vi "PROGRAM v0.96.vi"() -> ()   [LabVIEW 2015]
uses:
  <vilib>/Analysis/Matrix/Datatypes/RealMatrix.ctl
  <vilib>/DAQmx/write.llb/DAQmx Write (Digital 1D Bool 1Chan 1Samp).vi
  <vilib>/DAQmx/write.llb/DAQmx Write (Digital 1D Bool NChan 1Samp 1Line).vi
  <vilib>/DAQmx/read.llb/DAQmx Read (Analog Wfm 1Chan NSamp).vi
  <vilib>/DAQmx/write.llb/DAQmx Write (Analog 1D DBL NChan 1Samp).vi
  <vilib>/DAQmx/miscellaneous.llb/DAQmx Fill In Error Info.vi
  <vilib>/express/express analysis/Spectral/Block/exnSpectralBlock spectral measurements peak poly.vi
  <vilib>/express/express analysis/Spectral/Block/exnSpectralBlock spectral measurements peak WFM.vi
  <vilib>/express/express analysis/Spectral/XNode/ExpressSpectralMeasurementsBlockNode.xnode
  <vilib>/Analysis/Matrix/NI_Matrix.lvlib
panel:
  in  "Boolean":bool
  out "Kortslutningsström":dbl
  out "EQEvarv 2":i32
  in  "matrix":T1
  in  "Area":dbl caption="Frequency"
  out "Kortslutningsström frekvens":dbl
  in  "EQE-graf":enum32{"Sekvens-graf", "Frekvens-graf"}(tab)
  out "EQE sekvens graf":cluster{dbl[], ext[unit][]}(graph)
  out "EQE frekvens graf":cluster{dbl[], ext[unit][]}(graph)
  in  "stop":bool=TRUE
  in  "Ström från EQE-mätning":dbl[](array[numeric])
  in  "Reglage 720 nm":dbl(slide)=95.45983019683155 scale=0.0..100.0
  in  "Reglage 980 nm":dbl(slide)=100.00009164020905 scale=0.0..100.0
  in  "Reglage 830 nm":dbl(slide)=55.95186186163266 scale=0.0..100.0
  in  "Reglage 590 nm":dbl(slide)=99.99995581432673 scale=0.0..100.0
  in  "Reglage 515 nm":dbl(slide)=34.61040031085785 scale=0.0..100.0
  in  "Reglage 490 nm":dbl(slide)=100.00002446609867 scale=0.0..100.0
  in  "Reglage 750 nm":dbl(slide)=43.28879590477169 scale=0.0..100.0
  in  "Reglage 660 nm":dbl(slide)=45.024171978950314 scale=0.0..100.0
  in  "Reglage 630 nm":dbl(slide)=63.99528760647585 scale=0.0..100.0
  in  "Reglage 780 nm":dbl(slide)=34.69416555258395 scale=0.0..100.0
  in  "Reglage 450 nm":dbl(slide)=50.23408880646861 scale=0.0..100.0
  in  "Reglage 420 nm":dbl(slide)=37.90622795810308 caption="420 nm" scale=0.0..100.0 scale format="%3.0f"
  in  "Reglage 880 nm":dbl(slide)=65.6949904347887 scale=0.0..100.0
  in  "Reglage 945 nm":dbl(slide)=23.435133120769358 scale=0.0..100.0
  in  "Reglage 680 nm":dbl(slide)=85.53036777533312 scale=0.0..100.0
  in  "Reglage 520 nm":dbl(slide)=95.60915775479367 scale=0.0..100.0
  out "Kortslutnings-\nström":dbl
  out "Öppen krets-\nspänning":dbl
  out "PCE":dbl
  out "Fill factor":dbl format="%_6g"
  in  "Avsluta programmet":bool
  in  "Tänd/släck solen":bool
  out "EQEvarv":i32
  in  "Textfil":path
  in  "Val av EQE-mätning":enum32{"Sekvens", "Frekvens"}(radio)
  in  "Fördröjning/punkt (s)":dbl
  in  "Maximal ström":dbl=0.1
  in  "Frekvens (520 nm)":dbl caption="Frequency"
  out "IV-graf":cluster{"Voltage":sgl[], "Current":sgl[]}(graph)
  in  "Area":dbl caption="Frequency"
  in  "EQE-mätning":bool
  in  "IV-mätning":bool
  in  "Steglängd":dbl caption="Frequency"
  in  "Minspänning":dbl caption="Frequency"
  in  "Maxspänning":dbl caption="Frequency"
  in  "Alternativ":u16(ring)=2 items=["Ställ in värden manuellt", "Ställ in värden med reglage", "Standardspektrum AM1.5", "Nollställ alla intensiteter", "Maxa alla intensiteter", "Läs in spektrum från textfil"]
  in  "Intensitet (720)":dbl=40.363
  in  "Intensitet (980)":dbl=88.8364
  in  "Frekvens (720 nm)":dbl caption="Frequency"
  in  "Frekvens (980 nm)":dbl caption="Frequency"
  in  "Intensitet (830)":dbl=46.9522
  in  "Intensitet (590)":dbl=80.0856
  in  "Intensitet (515)":dbl=21.5524
  in  "Frekvens (830 nm)":dbl caption="Frequency"
  in  "Frekvens (590 nm)":dbl caption="Frequency"
  in  "Frekvens (515 nm)":dbl caption="Frequency"
  in  "Intensitet (490)":dbl=48.2735
  in  "Intensitet (750)":dbl=31.2257
  in  "Intensitet (660)":dbl=33.2227
  in  "Frekvens (490 nm)":dbl caption="Frequency"
  in  "Frekvens (750 nm)":dbl caption="Frequency"
  in  "Frekvens (660 nm)":dbl caption="Frequency"
  in  "Intensitet (630)":dbl=48.8157
  in  "Intensitet (780)":dbl=43.738
  in  "Frekvens (630 nm)":dbl caption="Frequency"
  in  "Frekvens (780 nm)":dbl caption="Frequency"
  in  "Intensitet (450)":dbl=50.5233
  in  "Intensitet (420)":dbl=40.9749
  in  "Intensitet (880)":dbl=49.2385
  in  "Frekvens (450 nm)":dbl caption="Frequency"
  in  "Frekvens (420 nm)":dbl caption="Frequency"
  in  "Frekvens (880 nm)":dbl caption="Frequency"
  in  "Intensitet (945)":dbl=21.9074
  in  "Intensitet (680)":dbl=38.1331
  in  "Intensitet (520)":dbl=56.6743
  in  "Andel intensitet för\nangivet spektrum":dbl(slide)=1.0 scale=0.0001..1.0
  in  "Frekvens (945 nm)":dbl caption="Frequency"
  in  "Frekvens (680 nm)":dbl caption="Frequency"
  # "Intensitet"
  # "420 nm"
  # "450 nm"
  # "490 nm"
  # "515 nm"
  # "520 nm"
  # "590 nm"
  # "630 nm"
  # "660 nm"
  # "Intensitet (W/m²)"
  # "Intensitet (W/m²)"
  # "Intensitet (W/m²)"
  # "Intensitet (W/m²)"
  # "Intensitet (W/m²)"
  # "Intensitet (W/m²)"
  # "Intensitet (W/m²)"
  # "Intensitet (W/m²)"
  # "680 nm"
  # "720 nm"
  # "750 nm"
  # "780 nm"
  # "830 nm"
  # "880 nm"
  # "945 nm"
  # "980 nm"
  # "Intensitet (W/m²)"
  # "Intensitet (W/m²)"
  # "Intensitet (W/m²)"
  # "Intensitet (W/m²)"
  # "Intensitet (W/m²)"
  # "Intensitet (W/m²)"
  # "Intensitet (W/m²)"
  # "Intensitet (W/m²)"
  # "Saker att göra:\n- ta loss fläkt och öka avståndet för att minska ljudet \n- mät homogenisering för alla färger (över 4x4cm^2 9 mätpunkter)\n- Verifiera AM1.5 med diod.\n- Verifiera AM1.5 med spektrometer.\n- Mäta på egna solceller.\n- Dokumentation på allt."
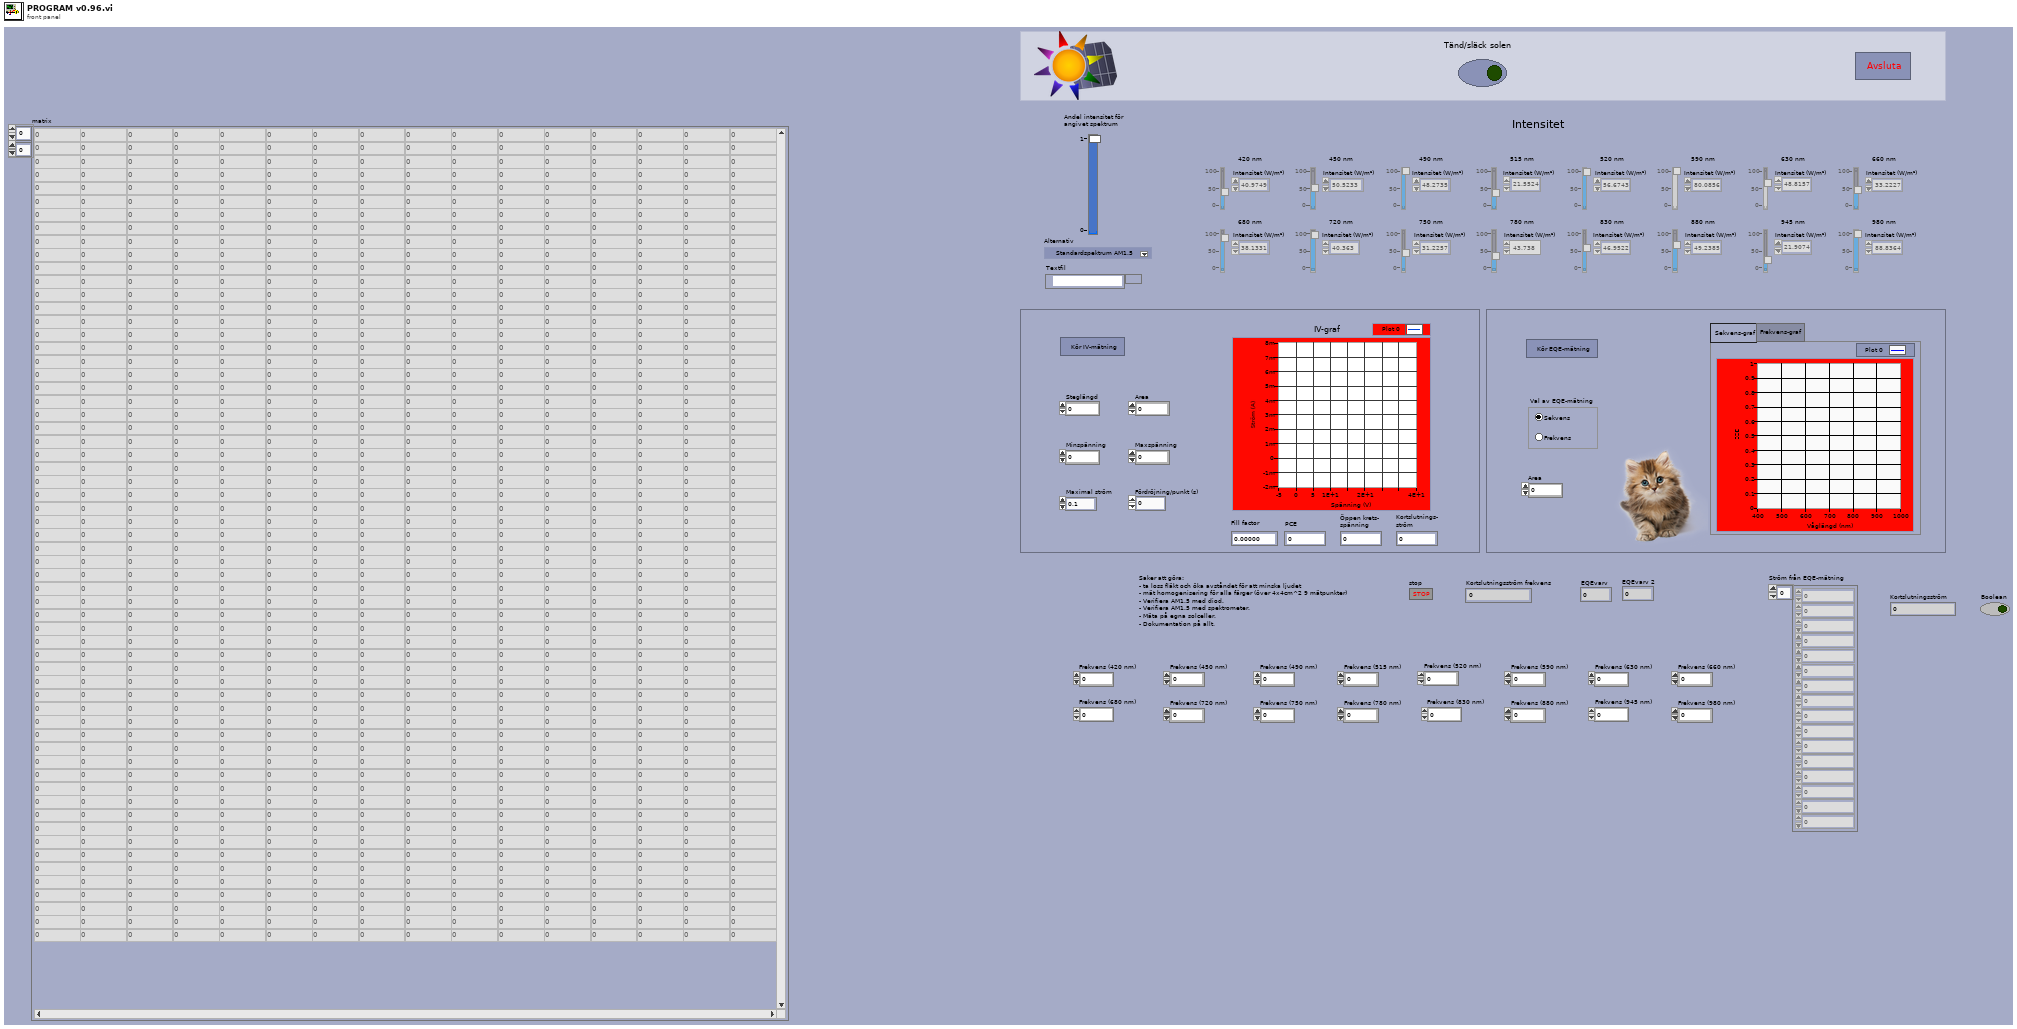
[diagram p1: front panel]
types:
  T1 = typedef "NI_Matrix.lvlib/RealMatrix.ctl" = dbl[][]
  T2 = enum8{"Enabled", "Disabled", "Disabled and Grayed Out"}
  T3 = cluster{"averaging mode":u16, "weighting mode":u16, "number of averages":u32}
  T4 = cluster{"dB On (F)":bool, "unwrap phase (F)":bool, "convert to degree (F)":bool}
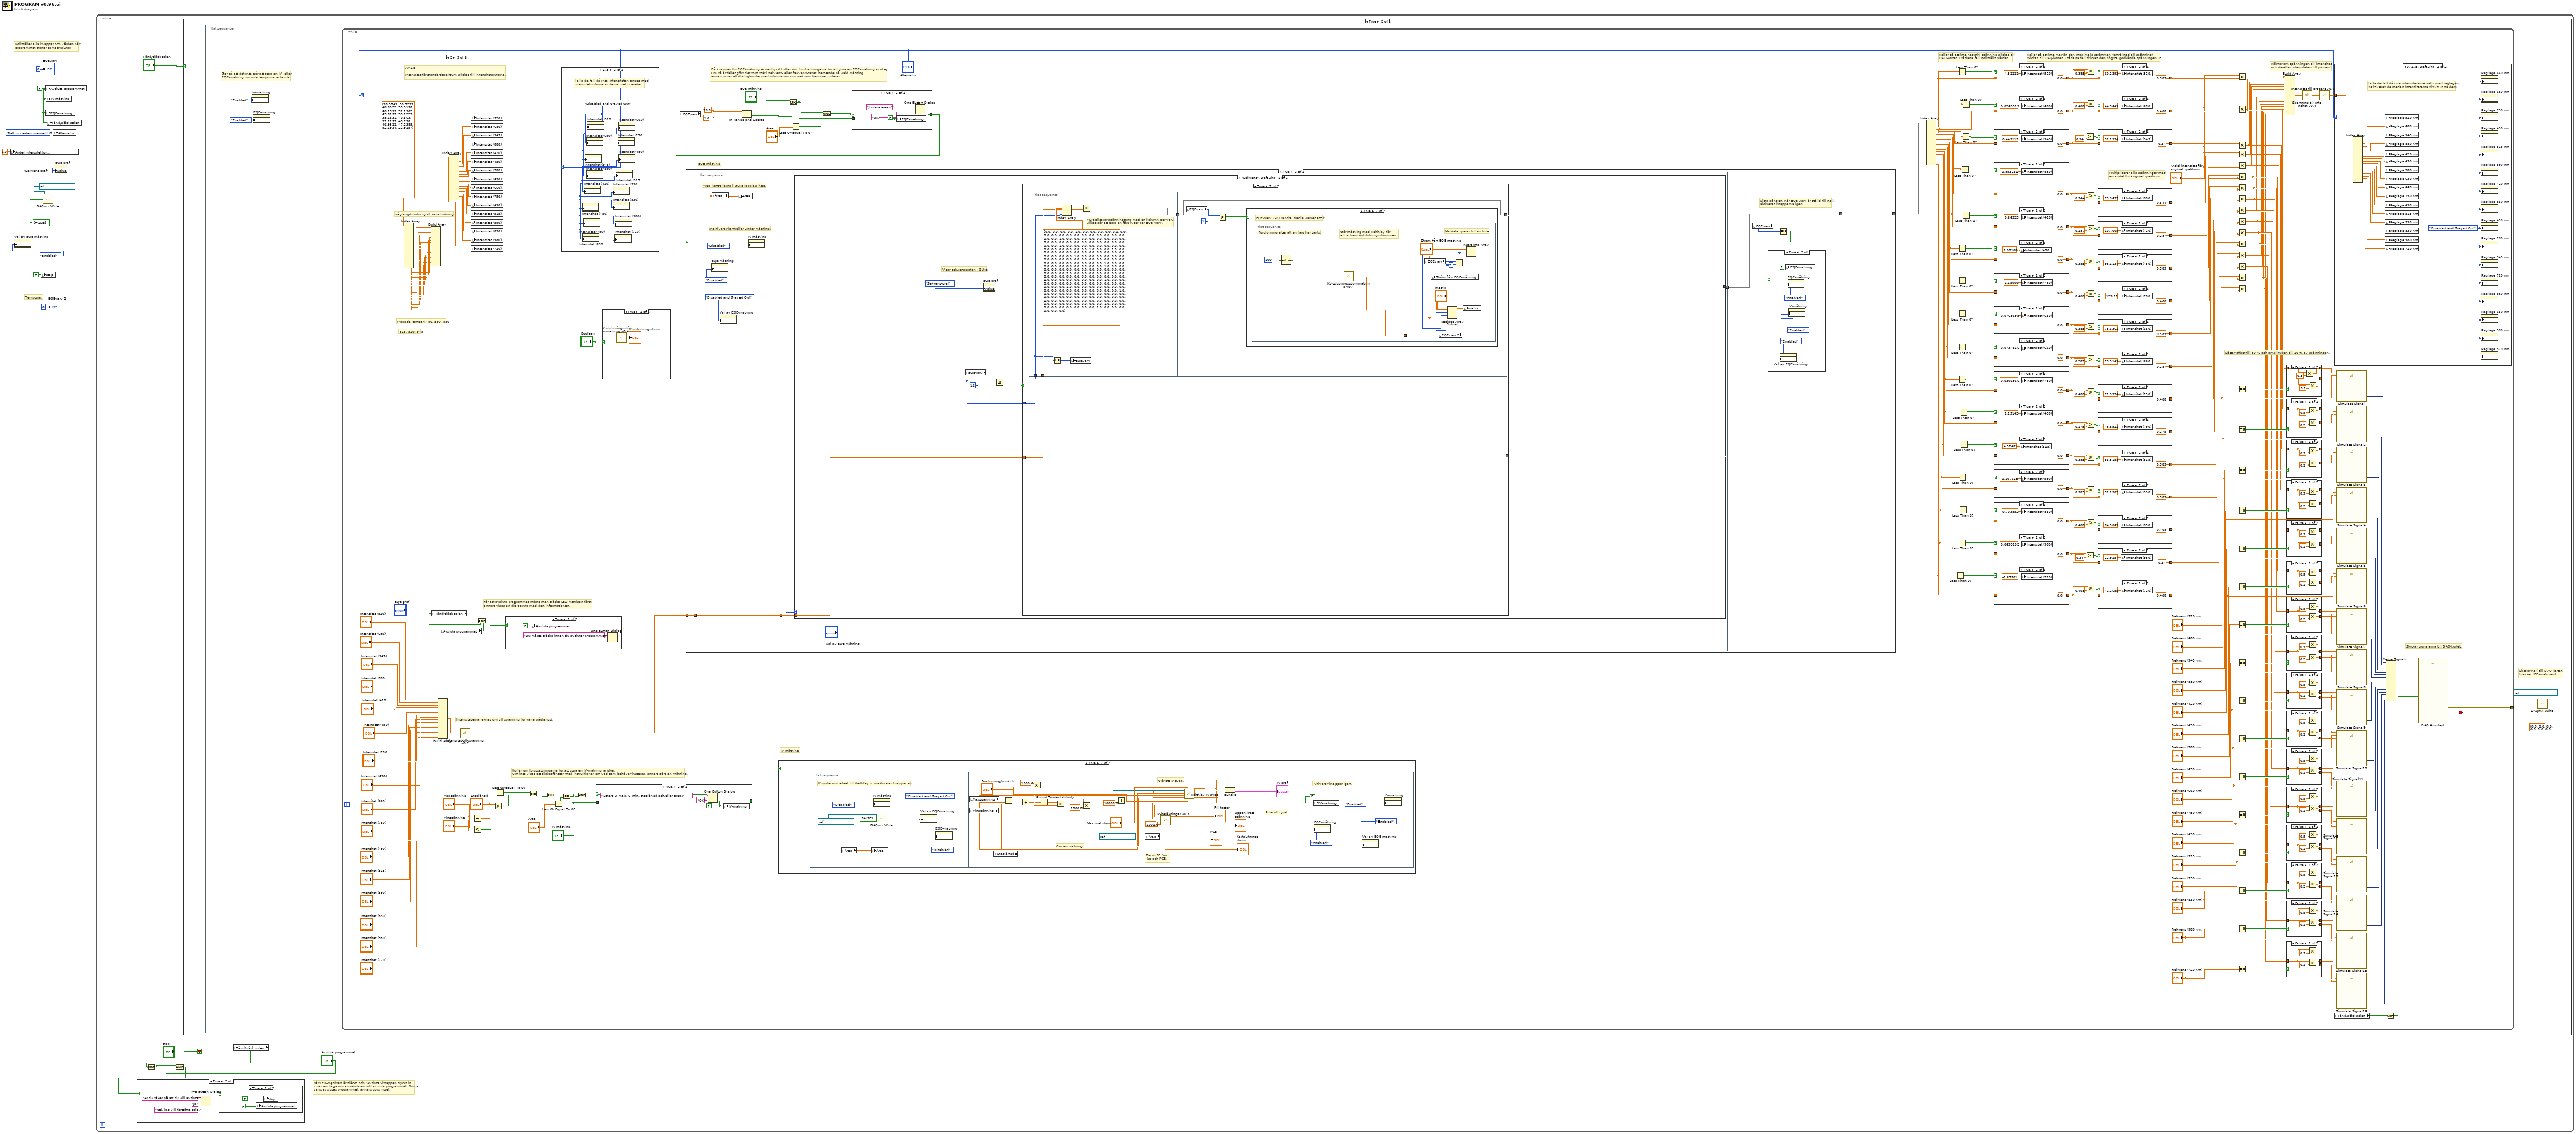
[diagram p0: block diagram]
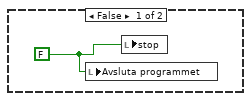
[diagram p3: hidden frame]
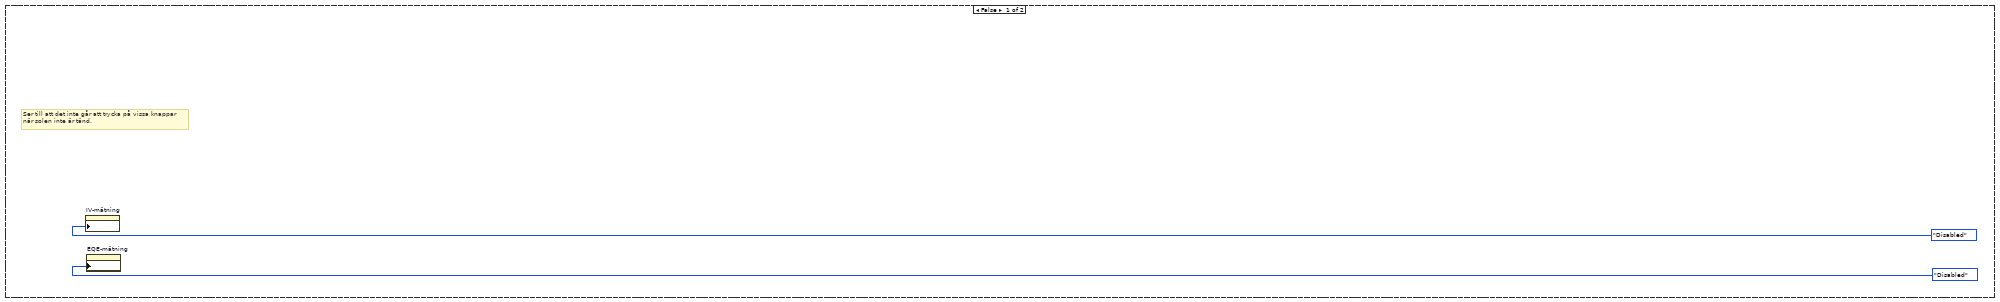
[diagram p4: hidden frame]
diagram:
  w8 = u16 0 items=["Ställ in värden manuellt", "Ställ in värden med reglage", "Standardspektrum AM1.5", "Nollställ alla frekvenser", "Nollställ alla spänningar", "Maxa alla spänningar", "Läs in spektrum från textfil"] ("Alternativ")
  w9 = FALSE ("Avsluta programmet")
  # "Temporär:"
  # "Nollställer alla knappar och värden när\nprogrammet startar samt avslutar."
  n1 = local write "Andel intensitet för\nangivet spektrum"(1.0 ("Andel intensitet för\nangivet spektrum")) -> ()
  n2 = property on="Val av EQE-mätning" class="RadioBtnsControl (strict)"("DisabledEnum"=T2."Enabled" ("Disabled")) -> ()  [unwired: 2 in, 2 out]
  n3 = local write "stop"(FALSE ("stop")) -> ()
  n4 = call-poly <vilib>:"DAQmx Write.vi"("task/channels in"=refnum<k21> "Reläomkoppling", "data"=bool[] [FALSE]) -> ()  [unwired: 11 in, 3 out]
  n5 = local write "Avsluta programmet"(w9) -> ()
  n6 = local write "EQE-mätning"(w9) -> ()
  n7 = local write "IV-mätning"(w9) -> ()
  n8 = local write "Tänd/släck solen"(w9) -> ()
  n9 = local write "Alternativ"(w8) -> ()
  n10 = property on="EQE-graf" class="TabCtl (strict)"("Value"=enum32{"Sekvens-graf", "Frekvens-graf"}."Sekvens-graf" ("EQE-graf")) -> ()  [unwired: 2 in, 2 out]
  n11 = while {
    stop <- "stop" stop-if-true
    # "När LED-matrisen är släckt, och \"Avsluta\"-knappen trycks in,\nvisas en fråga om användaren vill avsluta programmet. Om ja\nväljs avslutas programmet, annars görs inget."
    n12 = case shown="True" "Tänd/släck solen" {
      frame False {
        # "Ser till att det inte går att trycka på vissa knappar \nnär solen inte är tänd."
        n13 = property on="IV-mätning" class="Bool (strict)"("DisabledEnum"=T2."Disabled" ("Disabled")) -> ()  [unwired: 2 in, 2 out]
        n14 = property on="EQE-mätning" class="Bool (strict)"("DisabledEnum"=T2."Disabled" ("Disabled")) -> ()  [unwired: 2 in, 2 out]
      }
      frame True {
        n15 = flat-sequence {
          frame #0 {
            # "Gör så att det inte går att göra en IV- eller\nEQE-mätning om inte lamporna är tända."
            n16 = property on="IV-mätning" class="Bool (strict)"("DisabledEnum"=T2."Enabled" ("Disabled")) -> ()  [unwired: 2 in, 2 out]
            n17 = property on="EQE-mätning" class="Bool (strict)"("DisabledEnum"=T2."Enabled" ("Disabled")) -> ()  [unwired: 2 in, 2 out]
          }
          frame #1 {
            # "Skickar noll till DAQ-kortet\n(släcker LED-matrisen)."
            n18 = while {
              tunnel: [w144] -> w28
              stop <- w150 stop-if-true
              # "Skickar signalerna till DAQ-kortet."
              # "Sätter offset till 80 % och amplituden till 20 % av spänningen."
              # "Räknar om spänningen till intensitet\noch därefter intensiteten till procent."
              # "Multiplicerar alla spänningar med\nen andel för angivet spektrum."
              # "Kollar så att inte mer än den maximala strömmen (omräknad till spänning)\nskickas till DAQ-kortet. I sådana fall skickas den högsta godkända spänningen ut."
              # "Kollar så att inte negativ spänning skickas till\nDAQ-kortet. I sådana fall nollställs värdet."
              # "Kollar om förutsättningarna för att göra en IV-mätning är okej.\nOm inte visas ett dialogfönster med instruktioner om vad som behöver justeras, annars görs en mätning."
              # "IV-mätning"
              # "EQE-mätning"
              # "Då knappen för EQE-mätning är nedtryckt kollas om förutsättningarna för att göra en EQE-mätning är okej.\nOm så är fallet görs det som står i sekvens- eller frekvens-caset, beroende på vald mätning,\nannars visas ett dialogfönster med information om vad som behöver justeras."
              # "Intensiteterna räknas om till spänning för varje våglängd."
              # "För att avsluta programmet måste man släcka LED-matrisen först,\nannars visas en dialogruta med den informationen."
              n19 = case shown="2" "Alternativ" {
                frame 0, Default {
                  # "Intensiteterna anges med intensitetsrutorna."
                }
                frame 1 {
                  # "Reglage 450 nm"
                  # "Justera med reglagen.\n\nDe värden som står på intensitetsreglagen skickas till intensitetsrutorna."
                  n20 = Build Array("Reglage 420 nm", "Reglage 450 nm", "Reglage 490 nm", "Reglage 515 nm", "Reglage 520 nm", "Reglage 590 nm", "Reglage 630 nm", "Reglage 660 nm", "Reglage 680 nm", "Reglage 720 nm", "Reglage 750 nm", "Reglage 780 nm", "Reglage 830 nm", "Reglage 880 nm", "Reglage 945 nm", "Reglage 980 nm") -> (w405:dbl[])
                  n21 = call "Procent-till-intensitet v0.4.vi"("procent"=w405) -> ("intensitet"=w406:dbl[])
                  n22 = Index Array(array=w406) -> (element #1=w437:dbl, element #2=w435:dbl, element #3=w433:dbl, element #4=w431:dbl, element #5=w429:dbl, element #6=w427:dbl, element #7=w425:dbl, element #8=w423:dbl, element #9=w421:dbl, element #10=w419:dbl, element #11=w417:dbl, element #12=w415:dbl, element #13=w413:dbl, element #14=w411:dbl, element #15=w409:dbl, element #16=w407:dbl)  [unwired: 16 in]
                  n23 = property on="Intensitet (420)" class="DigNum (strict)"("Value"=w437) -> ()  [unwired: 2 in, 2 out]
                  n24 = property on="Intensitet (450)" class="DigNum (strict)"("Value"=w435) -> ()  [unwired: 2 in, 2 out]
                  n25 = property on="Intensitet (490)" class="DigNum (strict)"("Value"=w433) -> ()  [unwired: 2 in, 2 out]
                  n26 = property on="Intensitet (515)" class="DigNum (strict)"("Value"=w431) -> ()  [unwired: 2 in, 2 out]
                  n27 = property on="Intensitet (520)" class="DigNum (strict)"("Value"=w429) -> ()  [unwired: 2 in, 2 out]
                  n28 = property on="Intensitet (590)" class="DigNum (strict)"("Value"=w427) -> ()  [unwired: 2 in, 2 out]
                  n29 = property on="Intensitet (630)" class="DigNum (strict)"("Value"=w425) -> ()  [unwired: 2 in, 2 out]
                  n30 = property on="Intensitet (660)" class="DigNum (strict)"("Value"=w423) -> ()  [unwired: 2 in, 2 out]
                  n31 = property on="Intensitet (680)" class="DigNum (strict)"("Value"=w421) -> ()  [unwired: 2 in, 2 out]
                  n32 = property on="Intensitet (720)" class="DigNum (strict)"("Value"=w419) -> ()  [unwired: 2 in, 2 out]
                  n33 = property on="Intensitet (750)" class="DigNum (strict)"("Value"=w417) -> ()  [unwired: 2 in, 2 out]
                  n34 = property on="Intensitet (780)" class="DigNum (strict)"("Value"=w415) -> ()  [unwired: 2 in, 2 out]
                  n35 = property on="Intensitet (830)" class="DigNum (strict)"("Value"=w413) -> ()  [unwired: 2 in, 2 out]
                  n36 = property on="Intensitet (880)" class="DigNum (strict)"("Value"=w411) -> ()  [unwired: 2 in, 2 out]
                  n37 = property on="Intensitet (945)" class="DigNum (strict)"("Value"=w409) -> ()  [unwired: 2 in, 2 out]
                  n38 = property on="Intensitet (980)" class="DigNum (strict)"("Value"=w407) -> ()  [unwired: 2 in, 2 out]
                }
                frame 2 {
                  # "515, 520, 945"
                  # "Maxade lampor: 490, 590, 980"
                  # "våglängdsordning -> kanalordning"
                  # "AM1.5\n\nIntensitet för standardspektrum skickas till intensitetsrutorna."
                  n39 = Index Array(array=dbl[] [38.9749, 50.5233, 48.8522, 53.5158, 60.2393, 32.2302, 63.8157, 33.2227, 38.1331, 40.363, 31.2257, 43.738, 46.9522, 47.2385, 92.1934, 22.9257]) -> (element #1=w456:dbl, element #2=w455:dbl, element #3=w454:dbl, element #4=w453:dbl, element #5=w452:dbl, element #6=w451:dbl, element #7=w450:dbl, element #8=w449:dbl, element #9=w448:dbl, element #10=w447:dbl, element #11=w446:dbl, element #12=w445:dbl, element #13=w444:dbl, element #14=w443:dbl, element #15=w442:dbl, element #16=w441:dbl)  [unwired: 16 in]
                  n40 = Build Array(w452, w448, w442, w443, w456, w455, w445, w450, w449, w446, w454, w453, w451, w444, w441, w447) -> (w439:dbl[])
                  n41 = Index Array(array=w439) -> (element #1=w472:dbl, element #2=w471:dbl, element #3=w470:dbl, element #4=w469:dbl, element #5=w468:dbl, element #6=w467:dbl, element #7=w466:dbl, element #8=w465:dbl, element #9=w464:dbl, element #10=w463:dbl, element #11=w462:dbl, element #12=w461:dbl, element #13=w460:dbl, element #14=w459:dbl, element #15=w458:dbl, element #16=w457:dbl)  [unwired: 16 in]
                  n42 = local write "Intensitet (520)"(w472) -> ()
                  n43 = local write "Intensitet (680)"(w471) -> ()
                  n44 = local write "Intensitet (945)"(w470) -> ()
                  n45 = local write "Intensitet (880)"(w469) -> ()
                  n46 = local write "Intensitet (420)"(w468) -> ()
                  n47 = local write "Intensitet (450)"(w467) -> ()
                  n48 = local write "Intensitet (780)"(w466) -> ()
                  n49 = local write "Intensitet (630)"(w465) -> ()
                  n50 = local write "Intensitet (660)"(w464) -> ()
                  n51 = local write "Intensitet (750)"(w463) -> ()
                  n52 = local write "Intensitet (490)"(w462) -> ()
                  n53 = local write "Intensitet (515)"(w461) -> ()
                  n54 = local write "Intensitet (590)"(w460) -> ()
                  n55 = local write "Intensitet (830)"(w459) -> ()
                  n56 = local write "Intensitet (980)"(w458) -> ()
                  n57 = local write "Intensitet (720)"(w457) -> ()
                }
                frame 3 {
                  # "Nollställer spänningarna."
                  n58 = Index Array(array=dbl[] [4.52221, 0.0269513, 0.443111, -0.893231, 0.66323, 2.08108, 1.15006, 0.0769695, 0.0734316, 0.0301966, 2.25143, 4.52481, -0.107615, 0.703852, 0.0639202, -1.65501]) -> (element #1=w489:dbl, element #2=w488:dbl, element #3=w487:dbl, element #4=w486:dbl, element #5=w485:dbl, element #6=w484:dbl, element #7=w483:dbl, element #8=w482:dbl, element #9=w481:dbl, element #10=w480:dbl, element #11=w479:dbl, element #12=w478:dbl, element #13=w477:dbl, element #14=w476:dbl, element #15=w475:dbl, element #16=w474:dbl)  [unwired: 16 in]
                  n59 = local write "Intensitet (520)"(w489) -> ()
                  n60 = local write "Intensitet (680)"(w488) -> ()
                  n61 = local write "Intensitet (945)"(w487) -> ()
                  n62 = local write "Intensitet (880)"(w486) -> ()
                  n63 = local write "Intensitet (420)"(w485) -> ()
                  n64 = local write "Intensitet (450)"(w484) -> ()
                  n65 = local write "Intensitet (780)"(w483) -> ()
                  n66 = local write "Intensitet (630)"(w482) -> ()
                  n67 = local write "Intensitet (660)"(w481) -> ()
                  n68 = local write "Intensitet (750)"(w480) -> ()
                  n69 = local write "Intensitet (490)"(w479) -> ()
                  n70 = local write "Intensitet (515)"(w478) -> ()
                  n71 = local write "Intensitet (590)"(w477) -> ()
                  n72 = local write "Intensitet (830)"(w476) -> ()
                  n73 = local write "Intensitet (980)"(w475) -> ()
                  n74 = local write "Intensitet (720)"(w474) -> ()
                }
                frame 4 {
                  # "kanalordning -> våglängdsordning"
                  # "Maxar spänningarna."
                  n75 = Index Array(array=dbl[] [60.2393, 44.3649, 92.1934, 75.9657, 107.009, 98.1134, 123.12, 75.6362, 73.5149, 71.9374, 48.8522, 53.5158, 32.2302, 84.5063, 22.9257, 42.2655]) -> (element #1=w508:dbl, element #2=w509:dbl, element #3=w510:dbl, element #4=w511:dbl, element #5=w512:dbl, element #6=w513:dbl, element #7=w514:dbl, element #8=w515:dbl, element #9=w516:dbl, element #10=w517:dbl, element #11=w518:dbl, element #12=w519:dbl, element #13=w520:dbl, element #14=w521:dbl, element #15=w522:dbl, element #16=w523:dbl)  [unwired: 16 in]
                  n76 = Build Array(w512, w513, w518, w519, w508, w520, w515, w516, w509, w523, w517, w514, w521, w511, w510, w522) -> (w507:dbl[])
                  n77 = Index Array(array=w507) -> (element #1=w506:dbl, element #2=w505:dbl, element #3=w504:dbl, element #4=w503:dbl, element #5=w502:dbl, element #6=w501:dbl, element #7=w500:dbl, element #8=w499:dbl, element #9=w498:dbl, element #10=w497:dbl, element #11=w496:dbl, element #12=w495:dbl, element #13=w494:dbl, element #14=w493:dbl, element #15=w492:dbl, element #16=w491:dbl)  [unwired: 16 in]
                  n78 = local write "Intensitet (420)"(w506) -> ()
                  n79 = local write "Intensitet (450)"(w505) -> ()
                  n80 = local write "Intensitet (490)"(w504) -> ()
                  n81 = local write "Intensitet (515)"(w503) -> ()
                  n82 = local write "Intensitet (520)"(w502) -> ()
                  n83 = local write "Intensitet (590)"(w501) -> ()
                  n84 = local write "Intensitet (630)"(w500) -> ()
                  n85 = local write "Intensitet (660)"(w499) -> ()
                  n86 = local write "Intensitet (680)"(w498) -> ()
                  n87 = local write "Intensitet (720)"(w497) -> ()
                  n88 = local write "Intensitet (750)"(w496) -> ()
                  n89 = local write "Intensitet (780)"(w495) -> ()
                  n90 = local write "Intensitet (830)"(w494) -> ()
                  n91 = local write "Intensitet (880)"(w493) -> ()
                  n92 = local write "Intensitet (945)"(w492) -> ()
                  n93 = local write "Intensitet (980)"(w491) -> ()
                }
                frame 5 {
                  w538 = 22.9257 ("y")
                  w537 = 92.1934 ("y")
                  w536 = 75.9657 ("y")
                  w535 = 84.5063 ("y")
                  w534 = 123.12 ("y")
                  w533 = 71.9374 ("y")
                  w532 = 42.2655 ("y")
                  w531 = 44.3649 ("y")
                  w530 = 73.5149 ("y")
                  w529 = 75.6362 ("y")
                  w528 = 32.2302 ("y")
                  w527 = 60.2393 ("y")
                  w526 = 53.5158 ("y")
                  w525 = 48.8522 ("y")
                  w524 = 98.1134 ("y")
                  w539 = 107.009 ("y")
                  # "Om den inlästa intensiteten\när strörre än maxintensiteten\nskickas maxintensiteten ut istället."
                  # "Inläsning från textfil."
                  # "Output är intensitet i ordning\nefter stigande våglängd."
                  n94 = call "Read from file to 1D-array v0.2.vi"("file (use dialog)"="Textfil") -> ("appended array"=w573:dbl[], "new file path (Not A Path if cancelled)"=w572:path)
                  n95 = local write "Textfil"(w572) -> ()
                  n96 = Index Array(array=w573) -> (element #1=w555:dbl, element #2=w554:dbl, element #3=w553:dbl, element #4=w552:dbl, element #5=w551:dbl, element #6=w550:dbl, element #7=w549:dbl, element #8=w548:dbl, element #9=w547:dbl, element #10=w546:dbl, element #11=w545:dbl, element #12=w544:dbl, element #13=w543:dbl, element #14=w542:dbl, element #15=w541:dbl, element #16=w540:dbl)  [unwired: 16 in]
                  n97 = Greater?(x=w555, y=w539) -> (0:w571:bool)
                  n98 = Greater?(x=w554, y=w524) -> (0:w570:bool)
                  n99 = Greater?(x=w553, y=w525) -> (0:w569:bool)
                  n100 = Greater?(x=w552, y=w526) -> (0:w568:bool)
                  n101 = Greater?(x=w551, y=w527) -> (0:w564:bool)
                  n102 = Greater?(x=w550, y=w528) -> (0:w565:bool)
                  n103 = Greater?(x=w549, y=w529) -> (0:w566:bool)
                  n104 = Greater?(x=w548, y=w530) -> (0:w567:bool)
                  n105 = Greater?(x=w547, y=w531) -> (0:w556:bool)
                  n106 = Greater?(x=w546, y=w532) -> (0:w557:bool)
                  n107 = Greater?(x=w545, y=w533) -> (0:w558:bool)
                  n108 = Greater?(x=w544, y=w534) -> (0:w559:bool)
                  n109 = Greater?(x=w543, y=w535) -> (0:w563:bool)
                  n110 = Greater?(x=w542, y=w536) -> (0:w562:bool)
                  n111 = Greater?(x=w541, y=w537) -> (0:w561:bool)
                  n112 = Greater?(x=w540, y=w538) -> (0:w560:bool)
                  n113 = case shown="True" w571 {
                    tunnel: w555 -> [w605 _]
                    tunnel: w539 -> [_ w606]
                    frame False {
                      n114 = local write "Intensitet (420)"(w605) -> ()
                    }
                    frame True {
                      n115 = local write "Intensitet (420)"(w606) -> ()
                    }
                  }
                  n116 = case shown="True" w570 {
                    tunnel: w554 -> [w603 _]
                    tunnel: w524 -> [_ w604]
                    frame False {
                      n117 = local write "Intensitet (450)"(w603) -> ()
                    }
                    frame True {
                      n118 = local write "Intensitet (450)"(w604) -> ()
                    }
                  }
                  n119 = case shown="True" w569 {
                    tunnel: w553 -> [w601 _]
                    tunnel: w525 -> [_ w602]
                    frame False {
                      n120 = local write "Intensitet (490)"(w601) -> ()
                    }
                    frame True {
                      n121 = local write "Intensitet (490)"(w602) -> ()
                    }
                  }
                  n122 = case shown="True" w568 {
                    tunnel: w552 -> [w599 _]
                    tunnel: w526 -> [_ w600]
                    frame False {
                      n123 = local write "Intensitet (515)"(w599) -> ()
                    }
                    frame True {
                      n124 = local write "Intensitet (515)"(w600) -> ()
                    }
                  }
                  n125 = case shown="True" w564 {
                    tunnel: w551 -> [w597 _]
                    tunnel: w527 -> [_ w598]
                    frame False {
                      n126 = local write "Intensitet (520)"(w597) -> ()
                    }
                    frame True {
                      n127 = local write "Intensitet (520)"(w598) -> ()
                    }
                  }
                  n128 = case shown="True" w565 {
                    tunnel: w550 -> [w595 _]
                    tunnel: w528 -> [_ w596]
                    frame False {
                      n129 = local write "Intensitet (590)"(w595) -> ()
                    }
                    frame True {
                      n130 = local write "Intensitet (590)"(w596) -> ()
                    }
                  }
                  n131 = case shown="True" w566 {
                    tunnel: w549 -> [w593 _]
                    tunnel: w529 -> [_ w594]
                    frame False {
                      n132 = local write "Intensitet (630)"(w593) -> ()
                    }
                    frame True {
                      n133 = local write "Intensitet (630)"(w594) -> ()
                    }
                  }
                  n134 = case shown="True" w567 {
                    tunnel: w548 -> [w591 _]
                    tunnel: w530 -> [_ w592]
                    frame False {
                      n135 = local write "Intensitet (660)"(w591) -> ()
                    }
                    frame True {
                      n136 = local write "Intensitet (660)"(w592) -> ()
                    }
                  }
                  n137 = case shown="True" w556 {
                    tunnel: w547 -> [w589 _]
                    tunnel: w531 -> [_ w590]
                    frame False {
                      n138 = local write "Intensitet (680)"(w589) -> ()
                    }
                    frame True {
                      n139 = local write "Intensitet (680)"(w590) -> ()
                    }
                  }
                  n140 = case shown="True" w557 {
                    tunnel: w546 -> [w587 _]
                    tunnel: w532 -> [_ w588]
                    frame False {
                      n141 = local write "Intensitet (720)"(w587) -> ()
                    }
                    frame True {
                      n142 = local write "Intensitet (720)"(w588) -> ()
                    }
                  }
                  n143 = case shown="True" w558 {
                    tunnel: w545 -> [w585 _]
                    tunnel: w533 -> [_ w586]
                    frame False {
                      n144 = local write "Intensitet (750)"(w585) -> ()
                    }
                    frame True {
                      n145 = local write "Intensitet (750)"(w586) -> ()
                    }
                  }
                  n146 = case shown="True" w559 {
                    tunnel: w544 -> [w583 _]
                    tunnel: w534 -> [_ w584]
                    frame False {
                      n147 = local write "Intensitet (780)"(w583) -> ()
                    }
                    frame True {
                      n148 = local write "Intensitet (780)"(w584) -> ()
                    }
                  }
                  n149 = case shown="True" w563 {
                    tunnel: w543 -> [w581 _]
                    tunnel: w535 -> [_ w582]
                    frame False {
                      n150 = local write "Intensitet (830)"(w581) -> ()
                    }
                    frame True {
                      n151 = local write "Intensitet (830)"(w582) -> ()
                    }
                  }
                  n152 = case shown="True" w562 {
                    tunnel: w542 -> [w579 _]
                    tunnel: w536 -> [_ w580]
                    frame False {
                      n153 = local write "Intensitet (880)"(w579) -> ()
                    }
                    frame True {
                      n154 = local write "Intensitet (880)"(w580) -> ()
                    }
                  }
                  n155 = case shown="True" w561 {
                    tunnel: w541 -> [w577 _]
                    tunnel: w537 -> [_ w578]
                    frame False {
                      n156 = local write "Intensitet (945)"(w577) -> ()
                    }
                    frame True {
                      n157 = local write "Intensitet (945)"(w578) -> ()
                    }
                  }
                  n158 = case shown="True" w560 {
                    tunnel: w540 -> [w575 _]
                    tunnel: w538 -> [_ w576]
                    frame False {
                      n159 = local write "Intensitet (980)"(w575) -> ()
                    }
                    frame True {
                      n160 = local write "Intensitet (980)"(w576) -> ()
                    }
                  }
                }
              }
              n161 = local read "Tänd/släck solen"() -> (w140:bool)
              n162 = Build Array("Intensitet (520)", "Intensitet (680)", "Intensitet (945)", "Intensitet (880)", "Intensitet (420)", "Intensitet (450)", "Intensitet (780)", "Intensitet (630)", "Intensitet (660)", "Intensitet (750)", "Intensitet (490)", "Intensitet (515)", "Intensitet (590)", "Intensitet (830)", "Intensitet (980)", "Intensitet (720)") -> (w135:dbl[])
              n163 = local read "Avsluta programmet"() -> (w139:bool)
              n164 = call "Intensitet-till-spänning v0.7.vi"("Intensitet"=w135) -> ("Spänningar"=w65:dbl[])
              n165 = Subtract(x="Maxspänning", y="Minspänning") -> (x-y=w275:dbl)
              n166 = Less?(x="Maxspänning", y="Minspänning") -> (x < y?=w255:bool)
              n167 = And(x=w140, y=w139) -> (x .and. y?=w202:bool)
              n168 = Greater?(x="Steglängd", y=w275) -> (0:w273:bool)
              n169 = Less Or Equal To 0?(x="Steglängd") -> (x <= 0?=w35:bool)
              n170 = case shown="True" w202 {
                frame False {
                }
                frame True {
                  n171 = local write "Avsluta programmet"(FALSE ("Avsluta programmet")) -> ()
                  n172 = One Button Dialog(message="Du måste släcka innan du avslutar programmet.") -> ()  [unwired: 1 in, 1 out]
                }
              }
              n173 = Or(x=w35, y=w273) -> (x .or. y?=w274:bool)
              n174 = Or(x=w274, y=w255) -> (x .or. y?=w277:bool)
              n175 = Less Or Equal To 0?(x="Area") -> (x <= 0?=w36:bool)
              n176 = case shown="1..5" "Alternativ" {
                frame 0, Default {
                  w376 = T2."Enabled" ("Disabled")
                  # "I fallet då intensiteterna ställs in med\nintensitetsrutorna är dessa aktiverade."
                  n177 = property on="Intensitet (450)" class="DigNum (strict)"("DisabledEnum"=w376) -> ()  [unwired: 2 in, 2 out]
                  n178 = property on="Intensitet (630)" class="DigNum (strict)"("DisabledEnum"=w376) -> ()  [unwired: 2 in, 2 out]
                  n179 = property on="Intensitet (780)" class="DigNum (strict)"("DisabledEnum"=w376) -> ()  [unwired: 2 in, 2 out]
                  n180 = property on="Intensitet (420)" class="DigNum (strict)"("DisabledEnum"=w376) -> ()  [unwired: 2 in, 2 out]
                  n181 = property on="Intensitet (945)" class="DigNum (strict)"("DisabledEnum"=w376) -> ()  [unwired: 2 in, 2 out]
                  n182 = property on="Intensitet (680)" class="DigNum (strict)"("DisabledEnum"=w376) -> ()  [unwired: 2 in, 2 out]
                  n183 = property on="Intensitet (880)" class="DigNum (strict)"("DisabledEnum"=w376) -> ()  [unwired: 2 in, 2 out]
                  n184 = property on="Intensitet (520)" class="DigNum (strict)"("DisabledEnum"=w376) -> ()  [unwired: 2 in, 2 out]
                  n185 = property on="Intensitet (590)" class="DigNum (strict)"("DisabledEnum"=w376) -> ()  [unwired: 2 in, 2 out]
                  n186 = property on="Intensitet (830)" class="DigNum (strict)"("DisabledEnum"=w376) -> ()  [unwired: 2 in, 2 out]
                  n187 = property on="Intensitet (720)" class="DigNum (strict)"("DisabledEnum"=w376) -> ()  [unwired: 2 in, 2 out]
                  n188 = property on="Intensitet (980)" class="DigNum (strict)"("DisabledEnum"=w376) -> ()  [unwired: 2 in, 2 out]
                  n189 = property on="Intensitet (515)" class="DigNum (strict)"("DisabledEnum"=w376) -> ()  [unwired: 2 in, 2 out]
                  n190 = property on="Intensitet (750)" class="DigNum (strict)"("DisabledEnum"=w376) -> ()  [unwired: 2 in, 2 out]
                  n191 = property on="Intensitet (660)" class="DigNum (strict)"("DisabledEnum"=w376) -> ()  [unwired: 2 in, 2 out]
                  n192 = property on="Intensitet (490)" class="DigNum (strict)"("DisabledEnum"=w376) -> ()  [unwired: 2 in, 2 out]
                }
                frame 1..5 {
                  w377 = T2."Disabled and Grayed Out" ("Disabled")
                  # "I alla de fall då inte intensiteten anges med\nintensitetsrutorna är dessa inaktiverade."
                  n193 = property on="Intensitet (450)" class="DigNum (strict)"("DisabledEnum"=w377) -> ()  [unwired: 2 in, 2 out]
                  n194 = property on="Intensitet (630)" class="DigNum (strict)"("DisabledEnum"=w377) -> ()  [unwired: 2 in, 2 out]
                  n195 = property on="Intensitet (780)" class="DigNum (strict)"("DisabledEnum"=w377) -> ()  [unwired: 2 in, 2 out]
                  n196 = property on="Intensitet (420)" class="DigNum (strict)"("DisabledEnum"=w377) -> ()  [unwired: 2 in, 2 out]
                  n197 = property on="Intensitet (945)" class="DigNum (strict)"("DisabledEnum"=w377) -> ()  [unwired: 2 in, 2 out]
                  n198 = property on="Intensitet (680)" class="DigNum (strict)"("DisabledEnum"=w377) -> ()  [unwired: 2 in, 2 out]
                  n199 = property on="Intensitet (880)" class="DigNum (strict)"("DisabledEnum"=w377) -> ()  [unwired: 2 in, 2 out]
                  n200 = property on="Intensitet (520)" class="DigNum (strict)"("DisabledEnum"=w377) -> ()  [unwired: 2 in, 2 out]
                  n201 = property on="Intensitet (590)" class="DigNum (strict)"("DisabledEnum"=w377) -> ()  [unwired: 2 in, 2 out]
                  n202 = property on="Intensitet (830)" class="DigNum (strict)"("DisabledEnum"=w377) -> ()  [unwired: 2 in, 2 out]
                  n203 = property on="Intensitet (720)" class="DigNum (strict)"("DisabledEnum"=w377) -> ()  [unwired: 2 in, 2 out]
                  n204 = property on="Intensitet (980)" class="DigNum (strict)"("DisabledEnum"=w377) -> ()  [unwired: 2 in, 2 out]
                  n205 = property on="Intensitet (515)" class="DigNum (strict)"("DisabledEnum"=w377) -> ()  [unwired: 2 in, 2 out]
                  n206 = property on="Intensitet (750)" class="DigNum (strict)"("DisabledEnum"=w377) -> ()  [unwired: 2 in, 2 out]
                  n207 = property on="Intensitet (660)" class="DigNum (strict)"("DisabledEnum"=w377) -> ()  [unwired: 2 in, 2 out]
                  n208 = property on="Intensitet (490)" class="DigNum (strict)"("DisabledEnum"=w377) -> ()  [unwired: 2 in, 2 out]
                }
              }
              n209 = Or(x=w277, y=w36) -> (x .or. y?=w276:bool)
              n210 = And(x=w276, y="IV-mätning") -> (x .and. y?=w279:bool)
              n211 = case shown="True" w279 {
                tunnel: [w642 w643] -> w134
                tunnel: "IV-mätning" -> [w642 _]
                frame False {
                }
                frame True {
                  w643 = FALSE
                  n212 = One Button Dialog(message="Justera U_max, U_min, steglängd och/eller area!", button name ("OK")="OK") -> ()  [unwired: 1 out]
                  n213 = local write "IV-mätning"(w643) -> ()
                }
              }
              n214 = case shown="True" "Boolean" {
                frame False {
                }
                frame True {
                  n215 = call "Kortslutningsströmmätning v0.4.vi"() -> ("Kortslutningsström"=→"Kortslutningsström":dbl)
                }
              }
              n216 = local read "EQEvarv"() -> (w237:i32)
              n217 = In Range and Coerce(upper limit=18.0, x=w237, lower limit=1.0) -> (In Range?=w131:bool)  [unwired: 1 out]
              n218 = case shown="True" w134 {
                frame False {
                }
                frame True {
                  n219 = flat-sequence {
                    frame #0 {
                      # "Kopplar om reläet till Keithley:n, inaktiverar knappar etc."
                      n220 = local read "Area"() -> (w610:dbl)
                      n221 = local write "Area"(w610) -> ()
                      n222 = property on="IV-mätning" class="Bool (strict)"("DisabledEnum"=T2."Disabled" ("Disabled")) -> ()  [unwired: 2 in, 2 out]
                      n223 = call-poly <vilib>:"DAQmx Write.vi"("task/channels in"=refnum<k21> "Reläomkoppling", "data"=bool[] [FALSE]) -> ()  [unwired: 11 in, 3 out]
                      n224 = property on="Val av EQE-mätning" class="RadioBtnsControl (strict)"("DisabledEnum"=T2."Disabled and Grayed Out" ("Disabled")) -> ()  [unwired: 2 in, 2 out]
                      n225 = property on="EQE-mätning" class="Bool (strict)"("DisabledEnum"=T2."Disabled" ("Disabled")) -> ()  [unwired: 2 in, 2 out]
                    }
                    frame #1 {
                      # "Ritar ut i graf."
                      # "Tar ut FF, Voc,\n Jsc och PCE."
                      # "Gör ett IV-svep."
                      # "Gör en mätning."
                      n226 = local read "Maxspänning"() -> (w626:dbl)
                      n227 = local read "Minspänning"() -> (w627:dbl)
                      n228 = local read "Steglängd"() -> (w623:dbl)
                      n229 = Subtract(x=w626, y=w627) -> (x-y=w622:dbl)
                      n230 = Divide(x=w622, y=w623) -> (x/y=w624:dbl)
                      n231 = Multiply(x=1000.0, y="Fördröjning/punkt (s)") -> (x*y=w636:dbl)
                      n232 = Round Toward -Infinity(1:w624) -> (0:w629:dbl)
                      n233 = Multiply(x=w629, y=w636) -> (x*y=w630:dbl)
                      n234 = Multiply(x=w630, y=2000.0) -> (x*y=w633:dbl)
                      n235 = Add(x=w633, y=10000.0) -> (x+y=w632:dbl)
                      n236 = local read "Area"() -> (w620:dbl)
                      n237 = call "Keithley IV-svep.vi"("Timeout (10000 ms)"=w632, "Manual Settling Delay (0 sec)"="Fördröjning/punkt (s)", "Compliance  Level (0.1)"="Maximal ström", "Number of Points (5)"=w629, "Maximum Amplitude (2)"=w626, "Minimum Amplitude (1)"=w627, "VISA resource name"=refnum<visa-resource-name> "GPIB0::24::INSTR") -> ("Current"=w615:sgl[], "Voltage"=w613:sgl[])  [unwired: 2 in]
                      n238 = call "IV-beräkningar v0.3.vi"("Pin: utstrålad effekt/m2"=1000.0 ("Pin: utstrålad effekt/m"), "Solcellens area"=w620, "Ström"=w615, "Spänning"=w613) -> ("Kortslutningsström"=→"Kortslutnings-\nström":dbl, "Öppen krets-spänning"=→"Öppen krets-\nspänning":dbl, "PCE"=→"PCE":dbl, "Fill factor"=→"Fill factor":dbl)  [unwired: 4 in]
                      n239 = Bundle("Voltage"=w613, "Current"=w615) -> (→"IV-graf":cluster{"Voltage":sgl[], "Current":sgl[]})  [unwired: 1 in]
                    }
                    frame #2 {
                      # "Aktiverar knappar igen."
                      n240 = local write "IV-mätning"(FALSE) -> ()
                      n241 = property on="EQE-mätning" class="Bool (strict)"("DisabledEnum"=T2."Enabled" ("Disabled")) -> ()  [unwired: 2 in, 2 out]
                      n242 = property on="Val av EQE-mätning" class="RadioBtnsControl (strict)"("DisabledEnum"=T2."Enabled" ("Disabled")) -> ()  [unwired: 2 in, 2 out]
                      n243 = property on="IV-mätning" class="Bool (strict)"("DisabledEnum"=T2."Enabled" ("Disabled")) -> ()  [unwired: 2 in, 2 out]
                    }
                  }
                }
              }
              n244 = Or(x="EQE-mätning", y=w131) -> (x .or. y?=w67:bool)
              n245 = Less Or Equal To 0?(x="Area") -> (x <= 0?=w32:bool)
              n246 = And(x=w67, y=w32) -> (x .and. y?=w68:bool)
              n247 = case shown="True" w68 {
                tunnel: [w282 w283] -> w69
                tunnel: w67 -> [w282 _]
                frame False {
                }
                frame True {
                  w283 = FALSE
                  n248 = local write "EQE-mätning"(w283) -> ()
                  n249 = One Button Dialog(message="Justera arean!", button name ("OK")="OK") -> ()  [unwired: 1 out]
                }
              }
              n250 = case shown="True" w69 {
                tunnel: w65 -> [w646 w647]
                tunnel: [w646 w649] -> w146
                frame False {
                }
                frame True {
                  n251 = flat-sequence {
                    tunnel: w647 -> [w655]
                    tunnel: [w655] -> w648
                    tunnel: [w657] -> w650
                    tunnel: w648 -> [w658]
                    tunnel: [w949] -> w649
                    tunnel: w650 -> [w949]
                    frame #0 {
                      # "Inaktiverar kontroller under mätning."
                      # "Area-kontrollerna i GUI:t kopplas ihop."
                      n252 = property on="EQE-mätning" class="Bool (strict)"("DisabledEnum"=T2."Disabled" ("Disabled")) -> ()  [unwired: 2 in, 2 out]
                      n253 = local read "Area"() -> (w653:dbl)
                      n254 = property on="Val av EQE-mätning" class="RadioBtnsControl (strict)"("DisabledEnum"=T2."Disabled and Grayed Out" ("Disabled")) -> ()  [unwired: 2 in, 2 out]
                      n255 = local write "Area"(w653) -> ()
                      n256 = property on="IV-mätning" class="Bool (strict)"("DisabledEnum"=T2."Disabled" ("Disabled")) -> ()  [unwired: 2 in, 2 out]
                    }
                    frame #1 {
                      n257 = case shown="\"Sekvens\", Default" "Val av EQE-mätning" {
                        tunnel: w658 -> [w659 w755]
                        tunnel: [w662 w755] -> w657
                        frame "Sekvens", Default {
                          # "Visar sekvensgrafen i GUI:t."
                          n258 = local read "EQEvarv"() -> (w663:i32)
                          n259 = property on="EQE-graf" class="TabCtl (strict)"("Value"=enum32{"Sekvens-graf", "Frekvens-graf"}."Sekvens-graf" ("EQE-graf")) -> ()  [unwired: 2 in, 2 out]
                          n260 = Less Or Equal?(x=w663, y=16) -> (x <= y?=w661:bool)
                          n261 = case shown="True" w661 {
                            tunnel: w659 -> [w665 w729]
                            tunnel: [w665 w726] -> w662
                            tunnel: w663 -> [_ w728]
                            frame False {
                              n262 = flat-sequence {
                                frame #0 {
                                w666 = 1e-09 ("element")
                                w717 = ext[unit] 6.6260693000000000003e-34
                                w715 = ext[unit] 299792458.0
                                w719 = ext[unit] 1.60217652999999999996e-19
                                # "Ritar ut i graf."
                                # "Räknar ut EQE-värden för varje våglängd med hjälp av intensiteten, arean och den uppmätta strömmen."
                                n263 = local read "Andel intensitet för\nangivet spektrum"() -> (w671:dbl)
                                n264 = local read "Intensitet (420)"() -> (w693:dbl)
                                n265 = local read "Intensitet (450)"() -> (w692:dbl)
                                n266 = local read "Intensitet (490)"() -> (w691:dbl)
                                n267 = local read "Intensitet (515)"() -> (w690:dbl)
                                n268 = local read "Intensitet (520)"() -> (w689:dbl)
                                n269 = local read "Intensitet (590)"() -> (w688:dbl)
                                n270 = local read "Intensitet (630)"() -> (w687:dbl)
                                n271 = local read "Intensitet (660)"() -> (w686:dbl)
                                n272 = local read "Intensitet (680)"() -> (w685:dbl)
                                n273 = local read "Intensitet (720)"() -> (w684:dbl)
                                n274 = local read "Intensitet (750)"() -> (w683:dbl)
                                n275 = local read "Intensitet (780)"() -> (w682:dbl)
                                n276 = local read "Intensitet (830)"() -> (w681:dbl)
                                n277 = local read "Intensitet (880)"() -> (w680:dbl)
                                n278 = local read "Intensitet (945)"() -> (w679:dbl)
                                n279 = local read "Intensitet (980)"() -> (w678:dbl)
                                n280 = Build Array(420.0 ("element"), 450.0 ("element"), 490.0 ("element"), 515.0 ("element"), 520.0 ("element"), 590.0 ("element"), 630.0 ("element"), 660.0 ("element"), 680.0 ("element"), 720.0 ("element"), 750.0 ("element"), 780.0 ("element"), 830.0 ("element"), 880.0 ("element"), 945.0 ("element"), 980.0 ("element")) -> (w675:dbl[])
                                n281 = local read "Ström från EQE-mätning"() -> (w674:dbl[])
                                n282 = Build Array(w671, w671, w671, w671, w671, w671, w671, w671, w671, w671, w671, w671, w671, w671, w671, w671) -> (w668:dbl[])
                                n283 = Build Array(w693, w692, w691, w690, w689, w688, w687, w686, w685, w684, w683, w682, w681, w680, w679, w678) -> (w669:dbl[])
                                n284 = local read "Area"() -> (w722:dbl)
                                n285 = Build Array(w717, w717, w717, w717, w717, w717, w717, w717, w717, w717, w717, w717, w717, w717, w717, w717) -> (w718:ext[unit][])
                                n286 = Build Array(w715, w715, w715, w715, w715, w715, w715, w715, w715, w715, w715, w715, w715, w715, w715, w715) -> (w716:ext[unit][])
                                n287 = Build Array(w666, w666, w666, w666, w666, w666, w666, w666, w666, w666, w666, w666, w666, w666, w666, w666) -> (w667:dbl[])
                                n288 = Multiply(x=w668, y=w669) -> (x*y=w670:dbl[])
                                n289 = Multiply(x=w718, y=w716) -> (x*y=w714:ext[unit][])
                                n290 = Multiply(x=w675, y=w667) -> (x*y=w677:dbl[])
                                n291 = Build Array(w722, w722, w722, w722, w722, w722, w722, w722, w722, w722, w722, w722, w722, w722, w722, w722) -> (w721:dbl[])
                                n292 = Multiply(x=w721, y=w670) -> (x*y=w712:dbl[])
                                n293 = Divide(x=w714, y=w677) -> (x/y=w711:ext[unit][])
                                n294 = Build Array(w719, w719, w719, w719, w719, w719, w719, w719, w719, w719, w719, w719, w719, w719, w719, w719) -> (w720:ext[unit][])
                                n295 = Divide(x=w674, y=w720) -> (x/y=w713:ext[unit][])
                                n296 = Divide(x=w712, y=w711) -> (x/y=w710:ext[unit][])
                                n297 = Divide(x=w713, y=w710) -> (x/y=w673:ext[unit][])
                                n298 = Negate(x=w673) -> (-x=w672:ext[unit][])
                                n299 = Bundle(w675, w672) -> (→"EQE sekvens graf":cluster{dbl[], ext[unit][]})  [unwired: 1 in]
                                }
                                frame #1 {
                                # "Återställer EQE-varv till noll."
                                n300 = local read "EQEvarv 2"() -> (w724:i32)
                                n301 = local write "EQEvarv"(0 ("EQEvarv")) -> ()
                                n302 = Increment(x=w724) -> (x+1=w723:i32)
                                n303 = local write "EQEvarv 2"(w723) -> ()
                                }
                              }
                            }
                            frame True {
                              n304 = flat-sequence {
                                tunnel: w729 -> [w733]
                                tunnel: w728 -> [w730]
                                tunnel: [w732] -> w727
                                tunnel: [w736] -> w726
                                tunnel: w727 -> [w736]
                                frame #0 {
                                # "Multiplicerar spänningarna med en kolumn per varv,\nvilket gör att bara en färg lyser per EQE-varv."
                                n305 = Increment(x=w730) -> (x+1=w731:i32)
                                n306 = Index Array(array=T1 [[0.0, 0.0, 0.0, 0.0, 1.0, 0.0, 0.0, 0.0, 0.0, 0.0, 0.0, 0.0, 0.0, 0.0, 0.0, 0.0], [0.0, 0.0, 0.0, 0.0, 0.0, 0.0, 0.0, 0.0, 1.0, 0.0, 0.0, 0.0, 0.0, 0.0, 0.0, 0.0], [0.0, 0.0, 0.0, 0.0, 0.0, 0.0, 0.0, 0.0, 0.0, 0.0, 0.0, 0.0, 0.0, 0.0, 1.0, 0.0], [0.0, 0.0, 0.0, 0.0, 0.0, 0.0, 0.0, 0.0, 0.0, 0.0, 0.0, 0.0, 0.0, 1.0, 0.0, 0.0], [1.0, 0.0, 0.0, 0.0, 0.0, 0.0, 0.0, 0.0, 0.0, 0.0, 0.0, 0.0, 0.0, 0.0, 0.0, 0.0], [0.0, 1.0, 0.0, 0.0, 0.0, 0.0, 0.0, 0.0, 0.0, 0.0, 0.0, 0.0, 0.0, 0.0, 0.0, 0.0], [0.0, 0.0, 0.0, 0.0, 0.0, 0.0, 0.0, 0.0, 0.0, 0.0, 0.0, 1.0, 0.0, 0.0, 0.0, 0.0], [0.0, 0.0, 0.0, 0.0, 0.0, 0.0, 1.0, 0.0, 0.0, 0.0, 0.0, 0.0, 0.0, 0.0, 0.0, 0.0], [0.0, 0.0, 0.0, 0.0, 0.0, 0.0, 0.0, 1.0, 0.0, 0.0, 0.0, 0.0, 0.0, 0.0, 0.0, 0.0], [0.0, 0.0, 0.0, 0.0, 0.0, 0.0, 0.0, 0.0, 0.0, 0.0, 1.0, 0.0, 0.0, 0.0, 0.0, 0.0], [0.0, 0.0, 1.0, 0.0, 0.0, 0.0, 0.0, 0.0, 0.0, 0.0, 0.0, 0.0, 0.0, 0.0, 0.0, 0.0], [0.0, 0.0, 0.0, 1.0, 0.0, 0.0, 0.0, 0.0, 0.0, 0.0, 0.0, 0.0, 0.0, 0.0, 0.0, 0.0], [0.0, 0.0, 0.0, 0.0, 0.0, 1.0, 0.0, 0.0, 0.0, 0.0, 0.0, 0.0, 0.0, 0.0, 0.0, 0.0], [0.0, 0.0, 0.0, 0.0, 0.0, 0.0, 0.0, 0.0, 0.0, 0.0, 0.0, 0.0, 1.0, 0.0, 0.0, 0.0], [0.0, 0.0, 0.0, 0.0, 0.0, 0.0, 0.0, 0.0, 0.0, 0.0, 0.0, 0.0, 0.0, 0.0, 0.0, 1.0], [0.0, 0.0, 0.0, 0.0, 0.0, 0.0, 0.0, 0.0, 0.0, 1.0, 0.0, 0.0, 0.0, 0.0, 0.0, 0.0]] ("matrix"), index (col)=w730) -> (element=w734:dbl[])  [unwired: 1 in]
                                n307 = local write "EQEvarv"(w731) -> ()
                                n308 = Multiply(x=w734, y=w733) -> (x*y=w732:dbl[])
                                }
                                frame #1 {
                                n309 = local read "EQEvarv"() -> (w737:i32)
                                n310 = Greater?(x=w737, y=1) -> (0:w739:bool)
                                n311 = case shown="True" w739 {
                                frame False {
                                # "EQE-varv 1 (första varvet):\nGör ingenting. Skicka bara ut spänningen till dioderna med lägst våglängd och gå in på varv 1 igen."
                                }
                                frame True {
                                # "EQE-varv 2-17 (andra, tredje varvet etc.):"
                                n312 = flat-sequence {
                                tunnel: [w742] -> w740
                                tunnel: w740 -> [w743]
                                frame #0 {
                                # "Fördröjning efter att en färg har tänts."
                                n313 = Wait (ms)(milliseconds to wait=u32 100) -> ()  [unwired: 1 out]
                                }
                                frame #1 {
                                # "Gör mätning med Keithley för\natt ta fram kortslutningsströmmen."
                                n314 = call "Kortslutningsströmmätning v0.4.vi"() -> ("Kortslutningsström"=w742:dbl)
                                }
                                frame #2 {
                                # "Mätdata sparas till en lista."
                                n315 = local read "EQEvarv"() -> (w749:i32)
                                n316 = local read "EQEvarv 2"() -> (w744:i32)
                                n317 = Subtract(x=w749, y=2) -> (x-y=w747:i32)
                                n318 = Replace Array Subset(array="matrix", new element=w743, index (row)=w744, index (col)=w747) -> (w745:T1)
                                n319 = local write "matrix"(w745) -> ()
                                n320 = Insert Into Array(array="Ström från EQE-mätning", index=w747, new element=w743) -> (w750:dbl[])
                                n321 = local write "Ström från EQE-mätning"(w750) -> ()
                                }
                                }
                                }
                                }
                                }
                              }
                            }
                          }
                        }
                        frame "Frekvens" {
                          n322 = local read "EQEvarv"() -> (w753:i32)
                          n323 = Less Or Equal?(x=w753, y=1) -> (x <= y?=w754:bool)
                          n324 = case shown="False" w754 {
                            frame True {
                              n325 = flat-sequence {
                                frame #0 {
                                # "Första varvet i frekvensstyrda EQE-mätningen:\nKortslutningsströmmen mäts och ställer om reläerna\ni IV-konverteraren för att få rätt arbetsområde."
                                n326 = local read "EQEvarv"() -> (w757:i32)
                                n327 = Equal To 0?(x=w757) -> (x = 0?=w756:bool)
                                n328 = case shown="True" w756 {
                                frame False {
                                }
                                frame True {
                                n329 = call "Kortslutningsströmmätning v0.4.vi"() -> ("Kortslutningsström"=w759:dbl)
                                n330 = Absolute Value(x=w759) -> (abs(x)=w758:dbl)
                                "Kortslutningsström frekvens" <- w758
                                n331 = Less?(x=w758, y=0.01) -> (x < y?=w760:bool)
                                n332 = case shown="True" w760 {
                                tunnel: w758 -> [w764 _]
                                frame False {
                                n333 = Less?(x=w764, y=0.1) -> (x < y?=w762:bool)
                                n334 = case shown="True" w762 {
                                frame False {
                                n335 = call-poly <vilib>:"DAQmx Write.vi"("task/channels in"=refnum<k21> "Relädriftkretsomkoppling", "data"=bool[] [TRUE, TRUE]) -> ()  [unwired: 11 in, 3 out]
                                }
                                frame True {
                                n336 = call-poly <vilib>:"DAQmx Write.vi"("task/channels in"=refnum<k21> "Relädriftkretsomkoppling", "data"=bool[] [TRUE, FALSE]) -> ()  [unwired: 11 in, 3 out]
                                }
                                }
                                }
                                frame True {
                                n337 = call-poly <vilib>:"DAQmx Write.vi"("task/channels in"=refnum<k21> "Relädriftkretsomkoppling", "data"=bool[] [FALSE, FALSE]) -> ()  [unwired: 11 in, 3 out]
                                }
                                }
                                }
                                }
                                }
                                frame #1 {
                                w773 = 200.0
                                # "Visar frekvensgrafen i GUI:t."
                                # "Skickar ut intensiteterna med olika frekvenser."
                                n338 = Multiply(x=w773, y=1.0) -> (x*y=w806:dbl)
                                n339 = Multiply(x=w773, y=1.1) -> (x*y=w804:dbl)
                                n340 = Multiply(x=w773, y=1.2) -> (x*y=w802:dbl)
                                n341 = Multiply(x=w773, y=1.3) -> (x*y=w800:dbl)
                                n342 = Multiply(x=w773, y=1.4) -> (x*y=w798:dbl)
                                n343 = Multiply(x=w773, y=1.5) -> (x*y=w796:dbl)
                                n344 = Multiply(x=w773, y=1.6) -> (x*y=w794:dbl)
                                n345 = Multiply(x=w773, y=1.7) -> (x*y=w792:dbl)
                                n346 = Multiply(x=w773, y=1.05) -> (x*y=w805:dbl)
                                n347 = Multiply(x=w773, y=1.15) -> (x*y=w803:dbl)
                                n348 = Multiply(x=w773, y=1.25) -> (x*y=w801:dbl)
                                n349 = Multiply(x=w773, y=1.35) -> (x*y=w799:dbl)
                                n350 = Multiply(x=w773, y=1.45) -> (x*y=w797:dbl)
                                n351 = Multiply(x=w773, y=1.55) -> (x*y=w795:dbl)
                                n352 = Multiply(x=w773, y=1.65) -> (x*y=w793:dbl)
                                n353 = Multiply(x=w773, y=1.75) -> (x*y=w791:dbl)
                                n354 = local write "Frekvens (420 nm)"(w806) -> ()
                                n355 = local write "Frekvens (450 nm)"(w805) -> ()
                                n356 = local write "Frekvens (490 nm)"(w804) -> ()
                                n357 = local write "Frekvens (515 nm)"(w803) -> ()
                                n358 = local write "Frekvens (520 nm)"(w802) -> ()
                                n359 = local write "Frekvens (590 nm)"(w801) -> ()
                                n360 = local write "Frekvens (630 nm)"(w800) -> ()
                                n361 = local write "Frekvens (660 nm)"(w799) -> ()
                                n362 = local write "Frekvens (680 nm)"(w798) -> ()
                                n363 = local write "Frekvens (720 nm)"(w797) -> ()
                                n364 = local write "Frekvens (750 nm)"(w796) -> ()
                                n365 = local write "Frekvens (780 nm)"(w795) -> ()
                                n366 = local write "Frekvens (830 nm)"(w794) -> ()
                                n367 = local write "Frekvens (880 nm)"(w793) -> ()
                                n368 = local write "Frekvens (945 nm)"(w792) -> ()
                                n369 = local write "Frekvens (980 nm)"(w791) -> ()
                                n370 = local read "EQEvarv"() -> (w772:i32)
                                n371 = Increment(x=w772) -> (x+1=w771:i32)
                                n372 = property on="EQE-graf" class="TabCtl (strict)"("Value"=enum32{"Sekvens-graf", "Frekvens-graf"}."Frekvens-graf" ("EQE-graf")) -> ()  [unwired: 2 in, 2 out]
                                n373 = local write "EQEvarv"(w771) -> ()
                                }
                              }
                            }
                            frame False {
                              n374 = flat-sequence {
                                tunnel: [w810] -> w807
                                tunnel: w807 -> [w925]
                                frame #0 {
                                # "Kopplar om reläet till IV-konverteraren."
                                n375 = call-poly <vilib>:"DAQmx Write.vi"("task/channels in"=refnum<k21> "Reläomkoppling", "data"=bool[] [TRUE]) -> ()  [unwired: 11 in, 3 out]
                                }
                                frame #1 {
                                # "Fouriertransformerar mätdata."
                                # "Tar in mätdata från IV-konverteraren."
                                n376 = call-poly <vilib>:"DAQmx Read.vi"("task/channels in"=refnum<k21> "Indata från IV-konv frekvens") -> ("data"=w811:waveform(dbl))  [unwired: 12 in, 2 out]
                                n377 = xnode "Spectral Measurements"("Signals"=w811) -> ("FFT - (Peak)"=w810:cluster{"f0":dbl, "df":dbl, "magnitude":dbl[]})  [unwired: 1 in, 2 out]
                                }
                                frame #2 {
                                w823 = 1e-09
                                w834 = 0.2
                                w884 = ext[unit] 6.6260693000000000003e-34
                                w882 = ext[unit] 299792458.0
                                w886 = ext[unit] 1.60217652999999999996e-19
                                w923 = 200.0
                                # "Räknar utifrån strömmen, intensiteterna och\narean fram EQE-värdena för varje våglängd\noch ritar ut i en graf."
                                # "Delar på resistansen i IV-konverteraren för att få strömmen."
                                # "Skalar med 0.2 för\natt få hela spänningen."
                                # "Tar ut spänningen för varje\nvåglängd från fouriertransformen."
                                n378 = Unbundle(w925) -> ("df"=w921:dbl, "magnitude"=w835:dbl[])  [unwired: 1 out]
                                n379 = Build Array(w921, w921, w921, w921, w921, w921, w921, w921, w921, w921, w921, w921, w921, w921, w921, w921) -> (w919:dbl[])
                                n380 = Build Array(w923, w923, w923, w923, w923, w923, w923, w923, w923, w923, w923, w923, w923, w923, w923, w923) -> (w922:dbl[])
                                n381 = Multiply(x=dbl[] [1.0, 1.05, 1.1, 1.15, 1.2, 1.25, 1.3, 1.35, 1.4, 1.45, 1.5, 1.55, 1.6, 1.65, 1.7, 1.75] ("array"), y=w922) -> (x*y=w920:dbl[])
                                n382 = Divide(x=w920, y=w919) -> (x/y=w837:dbl[])
                                n383 = local read "Kortslutningsström frekvens"() -> (w840:dbl)
                                n384 = To Long Integer(number=w837) -> (32bit integer=w836:i32[])
                                n385 = Index Array(array=w836) -> (element #1=w830:i32, element #2=w918:i32, element #3=w917:i32, element #4=w916:i32, element #5=w915:i32, element #6=w914:i32, element #7=w913:i32, element #8=w912:i32, element #9=w911:i32, element #10=w910:i32, element #11=w909:i32, element #12=w908:i32, element #13=w907:i32, element #14=w906:i32, element #15=w905:i32, element #16=w904:i32)  [unwired: 16 in]
                                n386 = Index Array(array=w835, index #1=w830, index #2=w918, index #3=w917, index #4=w916, index #5=w915, index #6=w914, index #7=w913, index #8=w912, index #9=w911, index #10=w910, index #11=w909, index #12=w908, index #13=w907, index #14=w906, index #15=w905, index #16=w904) -> (element #1=w903:dbl, element #2=w831:dbl, element #3=w902:dbl, element #4=w901:dbl, element #5=w900:dbl, element #6=w899:dbl, element #7=w898:dbl, element #8=w897:dbl, element #9=w896:dbl, element #10=w895:dbl, element #11=w894:dbl, element #12=w893:dbl, element #13=w892:dbl, element #14=w891:dbl, element #15=w838:dbl, element #16=w890:dbl)
                                n387 = Build Array(w903, w831, w902, w901, w900, w899, w898, w897, w896, w895, w894, w893, w892, w891, w838, w890) -> (w832:dbl[])
                                n388 = Absolute Value(x=w840) -> (abs(x)=w839:dbl)
                                n389 = Build Array(w834, w834, w834, w834, w834, w834, w834, w834, w834, w834, w834, w834, w834, w834, w834, w834) -> (w833:dbl[])
                                n390 = Divide(x=w832, y=w833) -> (x/y=w825:dbl[])
                                n391 = Less?(x=w839, y=0.01) -> (x < y?=w842:bool)
                                n392 = case shown="False" w842 {
                                tunnel: w825 -> [w929 w939]
                                tunnel: [w926 w942] -> w841
                                tunnel: w839 -> [w928 _]
                                frame False {
                                n393 = Less?(x=w928, y=0.1) -> (x < y?=w927:bool)
                                n394 = case shown="False" w927 {
                                tunnel: w929 -> [w932 w936]
                                tunnel: [w931 w935] -> w926
                                frame False {
                                w934 = 0.838
                                n395 = Build Array(w934, w934, w934, w934, w934, w934, w934, w934, w934, w934, w934, w934, w934, w934, w934, w934) -> (w933:dbl[])
                                n396 = Divide(x=w932, y=w933) -> (x/y=w931:dbl[])
                                }
                                frame True {
                                w938 = 37.76
                                n397 = Build Array(w938, w938, w938, w938, w938, w938, w938, w938, w938, w938, w938, w938, w938, w938, w938, w938) -> (w937:dbl[])
                                n398 = Divide(x=w936, y=w937) -> (x/y=w935:dbl[])
                                }
                                }
                                }
                                frame True {
                                w941 = 417.1
                                n399 = Build Array(w941, w941, w941, w941, w941, w941, w941, w941, w941, w941, w941, w941, w941, w941, w941, w941) -> (w940:dbl[])
                                n400 = Divide(x=w939, y=w940) -> (x/y=w942:dbl[])
                                }
                                }
                                n401 = local read "Intensitet (420)"() -> (w860:dbl)
                                n402 = local read "Intensitet (450)"() -> (w859:dbl)
                                n403 = local read "Intensitet (490)"() -> (w858:dbl)
                                n404 = local read "Intensitet (515)"() -> (w857:dbl)
                                n405 = local read "Intensitet (520)"() -> (w856:dbl)
                                n406 = local read "Intensitet (590)"() -> (w855:dbl)
                                n407 = local read "Intensitet (630)"() -> (w854:dbl)
                                n408 = local read "Intensitet (660)"() -> (w853:dbl)
                                n409 = local read "Intensitet (680)"() -> (w852:dbl)
                                n410 = local read "Intensitet (720)"() -> (w851:dbl)
                                n411 = local read "Intensitet (750)"() -> (w850:dbl)
                                n412 = local read "Intensitet (780)"() -> (w849:dbl)
                                n413 = local read "Intensitet (830)"() -> (w848:dbl)
                                n414 = local read "Intensitet (880)"() -> (w847:dbl)
                                n415 = local read "Intensitet (945)"() -> (w846:dbl)
                                n416 = local read "Intensitet (980)"() -> (w845:dbl)
                                n417 = Build Array(w860, w859, w858, w857, w856, w855, w854, w853, w852, w851, w850, w849, w848, w847, w846, w845) -> (w844:dbl[])
                                n418 = Build Array(420.0 ("element"), 450.0 ("element"), 490.0 ("element"), 515.0 ("element"), 520.0 ("element"), 590.0 ("element"), 630.0 ("element"), 660.0 ("element"), 680.0 ("element"), 720.0 ("element"), 750.0 ("element"), 780.0 ("element"), 830.0 ("element"), 880.0 ("element"), 945.0 ("element"), 980.0 ("element")) -> (w828:dbl[])
                                n419 = local read "Area"() -> (w889:dbl)
                                n420 = Build Array(w884, w884, w884, w884, w884, w884, w884, w884, w884, w884, w884, w884, w884, w884, w884, w884) -> (w885:ext[unit][])
                                n421 = Build Array(w882, w882, w882, w882, w882, w882, w882, w882, w882, w882, w882, w882, w882, w882, w882, w882) -> (w883:ext[unit][])
                                n422 = Build Array(w823, w823, w823, w823, w823, w823, w823, w823, w823, w823, w823, w823, w823, w823, w823, w823) -> (w824:dbl[])
                                n423 = Build Array(w889, w889, w889, w889, w889, w889, w889, w889, w889, w889, w889, w889, w889, w889, w889, w889) -> (w888:dbl[])
                                n424 = Multiply(x=w885, y=w883) -> (x*y=w881:ext[unit][])
                                n425 = Multiply(x=w828, y=w824) -> (x*y=w829:dbl[])
                                n426 = Multiply(x=w888, y=w844) -> (x*y=w879:dbl[])
                                n427 = Divide(x=w881, y=w829) -> (x/y=w878:ext[unit][])
                                n428 = Build Array(w886, w886, w886, w886, w886, w886, w886, w886, w886, w886, w886, w886, w886, w886, w886, w886) -> (w887:ext[unit][])
                                n429 = Divide(x=w841, y=w887) -> (x/y=w880:ext[unit][])
                                n430 = Divide(x=w879, y=w878) -> (x/y=w877:ext[unit][])
                                n431 = Divide(x=w880, y=w877) -> (x/y=w826:ext[unit][])
                                n432 = Bundle(w828, w826) -> (→"EQE frekvens graf":cluster{dbl[], ext[unit][]})  [unwired: 1 in]
                                }
                                frame #3 {
                                w943 = 0.0
                                # "Återställer värden och kopplar tillbaka reläet till Keithley:n."
                                n433 = local write "EQEvarv"(0 ("EQEvarv")) -> ()
                                n434 = local write "Frekvens (420 nm)"(w943) -> ()
                                n435 = local write "Frekvens (450 nm)"(w943) -> ()
                                n436 = local write "Frekvens (490 nm)"(w943) -> ()
                                n437 = local write "Frekvens (515 nm)"(w943) -> ()
                                n438 = local write "Frekvens (520 nm)"(w943) -> ()
                                n439 = local write "Frekvens (590 nm)"(w943) -> ()
                                n440 = local write "Frekvens (630 nm)"(w943) -> ()
                                n441 = local write "Frekvens (660 nm)"(w943) -> ()
                                n442 = local write "Frekvens (680 nm)"(w943) -> ()
                                n443 = local write "Frekvens (720 nm)"(w943) -> ()
                                n444 = local write "Frekvens (750 nm)"(w943) -> ()
                                n445 = local write "Frekvens (780 nm)"(w943) -> ()
                                n446 = local write "Frekvens (830 nm)"(w943) -> ()
                                n447 = local write "Frekvens (880 nm)"(w943) -> ()
                                n448 = local write "Frekvens (945 nm)"(w943) -> ()
                                n449 = local write "Frekvens (980 nm)"(w943) -> ()
                                n450 = call-poly <vilib>:"DAQmx Write.vi"("task/channels in"=refnum<k21> "Reläomkoppling", "data"=bool[] [FALSE]) -> ()  [unwired: 11 in, 3 out]
                                }
                              }
                            }
                          }
                        }
                      }
                    }
                    frame #2 {
                      # "Sista gången, när EQE-varv är ställd till noll,\naktiveras knapparna igen."
                      n451 = local read "EQEvarv"() -> (w947:i32)
                      n452 = Equal To 0?(x=w947) -> (x = 0?=w948:bool)
                      n453 = case shown="True" w948 {
                        frame False {
                        }
                        frame True {
                          n454 = property on="Val av EQE-mätning" class="RadioBtnsControl (strict)"("DisabledEnum"=T2."Enabled" ("Disabled")) -> ()  [unwired: 2 in, 2 out]
                          n455 = local write "EQE-mätning"(FALSE ("EQE-mätning")) -> ()
                          n456 = property on="EQE-mätning" class="Bool (strict)"("DisabledEnum"=T2."Enabled" ("Disabled")) -> ()  [unwired: 2 in, 2 out]
                          n457 = property on="IV-mätning" class="Bool (strict)"("DisabledEnum"=T2."Enabled" ("Disabled")) -> ()  [unwired: 2 in, 2 out]
                        }
                      }
                    }
                  }
                }
              }
              n458 = Index Array(array=w146) -> (element #1=w236:dbl, element #2=w64:dbl, element #3=w62:dbl, element #4=w60:dbl, element #5=w59:dbl, element #6=w147:dbl, element #7=w56:dbl, element #8=w54:dbl, element #9=w52:dbl, element #10=w50:dbl, element #11=w48:dbl, element #12=w46:dbl, element #13=w44:dbl, element #14=w42:dbl, element #15=w40:dbl, element #16=w38:dbl)  [unwired: 16 in]
              n459 = Less Than 0?(x=w38) -> (x < 0?=w39:bool)
              n460 = Less Than 0?(x=w50) -> (x < 0?=w51:bool)
              n461 = Less Than 0?(x=w236) -> (x < 0?=w240:bool)
              n462 = Less Than 0?(x=w147) -> (x < 0?=w148:bool)
              n463 = Less Than 0?(x=w56) -> (x < 0?=w57:bool)
              n464 = Less Than 0?(x=w54) -> (x < 0?=w55:bool)
              n465 = Less Than 0?(x=w52) -> (x < 0?=w53:bool)
              n466 = Less Than 0?(x=w44) -> (x < 0?=w45:bool)
              n467 = Less Than 0?(x=w40) -> (x < 0?=w41:bool)
              n468 = Less Than 0?(x=w42) -> (x < 0?=w43:bool)
              n469 = Less Than 0?(x=w48) -> (x < 0?=w49:bool)
              n470 = Less Than 0?(x=w46) -> (x < 0?=w47:bool)
              n471 = Less Than 0?(x=w60) -> (x < 0?=w61:bool)
              n472 = Less Than 0?(x=w62) -> (x < 0?=w63:bool)
              n473 = Less Than 0?(x=w64) -> (x < 0?=w280:bool)
              n474 = Less Than 0?(x=w59) -> (x < 0?=w58:bool)
              n475 = case shown="True" w240 {
                tunnel: [w999 0.0 ("y")] -> w233
                tunnel: w236 -> [w999 _]
                frame False {
                }
                frame True {
                  n476 = local write "Intensitet (520)"(4.52221 ("Intensitet (520)")) -> ()
                }
              }
              n477 = case shown="True" w280 {
                tunnel: [w996 0.0 ("y")] -> w232
                tunnel: w64 -> [w996 _]
                frame False {
                }
                frame True {
                  n478 = local write "Intensitet (680)"(0.0269513 ("Spänning (520)")) -> ()
                }
              }
              n479 = case shown="True" w63 {
                tunnel: [w993 0.0 ("y")] -> w209
                tunnel: w62 -> [w993 _]
                frame False {
                }
                frame True {
                  n480 = local write "Intensitet (945)"(0.443111 ("Spänning (520)")) -> ()
                }
              }
              n481 = case shown="True" w61 {
                tunnel: [w990 0.0 ("y")] -> w207
                tunnel: w60 -> [w990 _]
                frame False {
                }
                frame True {
                  n482 = local write "Intensitet (880)"(-0.893231 ("Spänning (520)")) -> ()
                }
              }
              n483 = case shown="True" w58 {
                tunnel: [w987 0.0 ("y")] -> w212
                tunnel: w59 -> [w987 _]
                frame False {
                }
                frame True {
                  n484 = local write "Intensitet (420)"(0.66323 ("Spänning (520)")) -> ()
                }
              }
              n485 = case shown="True" w148 {
                tunnel: [w984 0.0 ("y")] -> w206
                tunnel: w147 -> [w984 _]
                frame False {
                }
                frame True {
                  n486 = local write "Intensitet (450)"(2.08108 ("Spänning (520)")) -> ()
                }
              }
              n487 = case shown="True" w57 {
                tunnel: [w981 0.0 ("y")] -> w205
                tunnel: w56 -> [w981 _]
                frame False {
                }
                frame True {
                  n488 = local write "Intensitet (780)"(1.15006 ("Spänning (520)")) -> ()
                }
              }
              n489 = case shown="True" w55 {
                tunnel: [w978 0.0 ("y")] -> w216
                tunnel: w54 -> [w978 _]
                frame False {
                }
                frame True {
                  n490 = local write "Intensitet (630)"(0.0769695 ("Spänning (520)")) -> ()
                }
              }
              n491 = case shown="True" w53 {
                tunnel: [w975 0.0 ("y")] -> w218
                tunnel: w52 -> [w975 _]
                frame False {
                }
                frame True {
                  n492 = local write "Intensitet (660)"(0.0734316 ("Spänning (520)")) -> ()
                }
              }
              n493 = case shown="True" w51 {
                tunnel: [w972 0.0 ("y")] -> w220
                tunnel: w50 -> [w972 _]
                frame False {
                }
                frame True {
                  n494 = local write "Intensitet (750)"(0.0301966 ("Spänning (520)")) -> ()
                }
              }
              n495 = case shown="True" w49 {
                tunnel: [w969 0.0 ("y")] -> w204
                tunnel: w48 -> [w969 _]
                frame False {
                }
                frame True {
                  n496 = local write "Intensitet (490)"(2.25143 ("Spänning (520)")) -> ()
                }
              }
              n497 = case shown="True" w47 {
                tunnel: [w966 0.0 ("y")] -> w223
                tunnel: w46 -> [w966 _]
                frame False {
                }
                frame True {
                  n498 = local write "Intensitet (515)"(4.52481 ("Spänning (520)")) -> ()
                }
              }
              n499 = case shown="True" w45 {
                tunnel: [w963 0.0 ("y")] -> w225
                tunnel: w44 -> [w963 _]
                frame False {
                }
                frame True {
                  n500 = local write "Intensitet (590)"(-0.107615 ("Spänning (520)")) -> ()
                }
              }
              n501 = case shown="True" w43 {
                tunnel: [w960 0.0 ("y")] -> w203
                tunnel: w42 -> [w960 _]
                frame False {
                }
                frame True {
                  n502 = local write "Intensitet (830)"(0.703852 ("Spänning (520)")) -> ()
                }
              }
              n503 = case shown="True" w41 {
                tunnel: [w957 0.0 ("y")] -> w228
                tunnel: w40 -> [w957 _]
                frame False {
                }
                frame True {
                  n504 = local write "Intensitet (980)"(0.0639202 ("Spänning (520)")) -> ()
                }
              }
              n505 = case shown="True" w39 {
                tunnel: [w954 0.0 ("y")] -> w230
                tunnel: w38 -> [w954 _]
                frame False {
                }
                frame True {
                  n506 = local write "Intensitet (720)"(-1.65501 ("Spänning (520)")) -> ()
                }
              }
              n507 = Greater?(x=w209, y=0.34) -> (0:w208:bool)
              n508 = Greater?(x=w228, y=0.34) -> (0:w227:bool)
              n509 = Greater?(x=w233, y=0.385) -> (0:w234:bool)
              n510 = Greater?(x=w232, y=0.408) -> (0:w231:bool)
              n511 = Greater?(x=w207, y=0.344) -> (0:w210:bool)
              n512 = Greater?(x=w212, y=0.287) -> (0:w211:bool)
              n513 = Greater?(x=w206, y=0.385) -> (0:w213:bool)
              n514 = Greater?(x=w205, y=0.408) -> (0:w214:bool)
              n515 = Greater?(x=w216, y=0.385) -> (0:w215:bool)
              n516 = Greater?(x=w218, y=0.287) -> (0:w217:bool)
              n517 = Greater?(x=w220, y=0.408) -> (0:w219:bool)
              n518 = Greater?(x=w204, y=0.275) -> (0:w221:bool)
              n519 = Greater?(x=w223, y=0.385) -> (0:w222:bool)
              n520 = Greater?(x=w225, y=0.385) -> (0:w224:bool)
              n521 = Greater?(x=w203, y=0.408) -> (0:w226:bool)
              n522 = Greater?(x=w230, y=0.408) -> (0:w229:bool)
              n523 = case shown="True" w234 {
                tunnel: w233 -> [w1047 _]
                tunnel: [w1047 0.385 ("y")] -> w154
                frame False {
                }
                frame True {
                  n524 = local write "Intensitet (520)"(60.2393 ("Intensitet (520)")) -> ()
                }
              }
              n525 = case shown="True" w231 {
                tunnel: w232 -> [w1044 _]
                tunnel: [w1044 0.408 ("y")] -> w200
                frame False {
                }
                frame True {
                  n526 = local write "Intensitet (680)"(44.3649 ("Intensitet (680)")) -> ()
                }
              }
              n527 = case shown="True" w208 {
                tunnel: w209 -> [w1041 _]
                tunnel: [w1041 0.34 ("y")] -> w155
                frame False {
                }
                frame True {
                  n528 = local write "Intensitet (945)"(92.1934 ("Intensitet (945)")) -> ()
                }
              }
              n529 = case shown="True" w210 {
                tunnel: w207 -> [w1038 _]
                tunnel: [w1038 0.344 ("y")] -> w199
                frame False {
                }
                frame True {
                  n530 = local write "Intensitet (880)"(75.9657 ("Intensitet (880)")) -> ()
                }
              }
              n531 = case shown="True" w211 {
                tunnel: w212 -> [w1035 _]
                tunnel: [w1035 0.287 ("y")] -> w156
                frame False {
                }
                frame True {
                  n532 = local write "Intensitet (420)"(107.009 ("Intensitet (420)")) -> ()
                }
              }
              n533 = case shown="True" w213 {
                tunnel: w206 -> [w1032 _]
                tunnel: [w1032 0.385 ("y")] -> w198
                frame False {
                }
                frame True {
                  n534 = local write "Intensitet (450)"(98.1134 ("Intensitet (450)")) -> ()
                }
              }
              n535 = case shown="True" w214 {
                tunnel: w205 -> [w1029 _]
                tunnel: [w1029 0.408 ("y")] -> w197
                frame False {
                }
                frame True {
                  n536 = local write "Intensitet (780)"(123.12 ("Intensitet (780)")) -> ()
                }
              }
              n537 = case shown="True" w215 {
                tunnel: w216 -> [w1026 _]
                tunnel: [w1026 0.385 ("y")] -> w157
                frame False {
                }
                frame True {
                  n538 = local write "Intensitet (630)"(75.6362 ("Intensitet (630)")) -> ()
                }
              }
              n539 = case shown="True" w217 {
                tunnel: w218 -> [w1023 _]
                tunnel: [w1023 0.287 ("y")] -> w158
                frame False {
                }
                frame True {
                  n540 = local write "Intensitet (660)"(73.5149 ("Intensitet (660)")) -> ()
                }
              }
              n541 = case shown="True" w219 {
                tunnel: w220 -> [w1020 _]
                tunnel: [w1020 0.408 ("y")] -> w159
                frame False {
                }
                frame True {
                  n542 = local write "Intensitet (750)"(71.9374 ("Intensitet (750)")) -> ()
                }
              }
              n543 = case shown="True" w221 {
                tunnel: w204 -> [w1017 _]
                tunnel: [w1017 0.275 ("y")] -> w196
                frame False {
                }
                frame True {
                  n544 = local write "Intensitet (490)"(48.8522 ("Intensitet (490)")) -> ()
                }
              }
              n545 = case shown="True" w222 {
                tunnel: w223 -> [w1014 _]
                tunnel: [w1014 0.385 ("y")] -> w160
                frame False {
                }
                frame True {
                  n546 = local write "Intensitet (515)"(53.5158 ("Intensitet (515)")) -> ()
                }
              }
              n547 = case shown="True" w224 {
                tunnel: w225 -> [w1011 _]
                tunnel: [w1011 0.385 ("y")] -> w161
                frame False {
                }
                frame True {
                  n548 = local write "Intensitet (590)"(32.2302 ("Intensitet (590)")) -> ()
                }
              }
              n549 = case shown="True" w226 {
                tunnel: w203 -> [w1008 _]
                tunnel: [w1008 0.408 ("y")] -> w195
                frame False {
                }
                frame True {
                  n550 = local write "Intensitet (830)"(84.5063 ("Intensitet (830)")) -> ()
                }
              }
              n551 = case shown="True" w227 {
                tunnel: w228 -> [w1005 _]
                tunnel: [w1005 0.34 ("y")] -> w194
                frame False {
                }
                frame True {
                  n552 = local write "Intensitet (980)"(22.9257 ("Intensitet (980)")) -> ()
                }
              }
              n553 = case shown="True" w229 {
                tunnel: w230 -> [w1002 _]
                tunnel: [w1002 0.408 ("y")] -> w162
                frame False {
                }
                frame True {
                  n554 = local write "Intensitet (720)"(42.2655 ("Intensitet (720)")) -> ()
                }
              }
              n555 = Multiply(x="Andel intensitet för\nangivet spektrum", y=w154) -> (x*y=w143:dbl)
              n556 = Multiply(x="Andel intensitet för\nangivet spektrum", y=w200) -> (x*y=w128:dbl)
              n557 = Multiply(x=w155, y="Andel intensitet för\nangivet spektrum") -> (x*y=w124:dbl)
              n558 = Multiply(x="Andel intensitet för\nangivet spektrum", y=w199) -> (x*y=w120:dbl)
              n559 = Multiply(x=w156, y="Andel intensitet för\nangivet spektrum") -> (x*y=w116:dbl)
              n560 = Multiply(x=w198, y="Andel intensitet för\nangivet spektrum") -> (x*y=w112:dbl)
              n561 = Multiply(x=w197, y="Andel intensitet för\nangivet spektrum") -> (x*y=w108:dbl)
              n562 = Multiply(x=w157, y="Andel intensitet för\nangivet spektrum") -> (x*y=w104:dbl)
              n563 = Multiply(x=w158, y="Andel intensitet för\nangivet spektrum") -> (x*y=w101:dbl)
              n564 = Multiply(x=w159, y="Andel intensitet för\nangivet spektrum") -> (x*y=w97:dbl)
              n565 = Multiply(x=w196, y="Andel intensitet för\nangivet spektrum") -> (x*y=w93:dbl)
              n566 = Multiply(x=w160, y="Andel intensitet för\nangivet spektrum") -> (x*y=w89:dbl)
              n567 = Multiply(x=w161, y="Andel intensitet för\nangivet spektrum") -> (x*y=w85:dbl)
              n568 = Multiply(x=w195, y="Andel intensitet för\nangivet spektrum") -> (x*y=w81:dbl)
              n569 = Multiply(x=w194, y="Andel intensitet för\nangivet spektrum") -> (x*y=w74:dbl)
              n570 = Multiply(x=w162, y="Andel intensitet för\nangivet spektrum") -> (x*y=w73:dbl)
              n571 = Equal To 0?(x="Frekvens (520 nm)") -> (x = 0?=w272:bool)
              n572 = Equal To 0?(x="Frekvens (680 nm)") -> (x = 0?=w129:bool)
              n573 = Equal To 0?(x="Frekvens (945 nm)") -> (x = 0?=w125:bool)
              n574 = Equal To 0?(x="Frekvens (880 nm)") -> (x = 0?=w121:bool)
              n575 = Equal To 0?(x="Frekvens (420 nm)") -> (x = 0?=w117:bool)
              n576 = Equal To 0?(x="Frekvens (450 nm)") -> (x = 0?=w113:bool)
              n577 = Equal To 0?(x="Frekvens (780 nm)") -> (x = 0?=w109:bool)
              n578 = Equal To 0?(x="Frekvens (630 nm)") -> (x = 0?=w105:bool)
              n579 = Equal To 0?(x="Frekvens (660 nm)") -> (x = 0?=w100:bool)
              n580 = Equal To 0?(x="Frekvens (750 nm)") -> (x = 0?=w96:bool)
              n581 = Equal To 0?(x="Frekvens (490 nm)") -> (x = 0?=w92:bool)
              n582 = Equal To 0?(x="Frekvens (515 nm)") -> (x = 0?=w88:bool)
              n583 = Equal To 0?(x="Frekvens (590 nm)") -> (x = 0?=w84:bool)
              n584 = Equal To 0?(x="Frekvens (830 nm)") -> (x = 0?=w80:bool)
              n585 = Equal To 0?(x="Frekvens (980 nm)") -> (x = 0?=w75:bool)
              n586 = Equal To 0?(x="Frekvens (720 nm)") -> (x = 0?=w72:bool)
              n587 = Build Array(w143, w128, w124, w120, w116, w112, w108, w104, w101, w97, w93, w89, w85, w81, w74, w73) -> (w138:dbl[])
              n588 = case shown="False" w272 {
                tunnel: w143 -> [w398 w402]
                tunnel: [w400 w402] -> w177
                tunnel: [w397 w402] -> w130
                frame False {
                  n589 = Multiply(x=w398, y=0.5) -> (x*y=w400:dbl)
                  n590 = Multiply(x=w398, y=0.2) -> (x*y=w397:dbl)
                }
                frame True {
                }
              }
              n591 = case shown="False" w129 {
                tunnel: w128 -> [w371 w375]
                tunnel: [w373 w375] -> w127
                tunnel: [w370 w375] -> w126
                frame False {
                  n592 = Multiply(x=w371, y=0.5) -> (x*y=w373:dbl)
                  n593 = Multiply(x=w371, y=0.2) -> (x*y=w370:dbl)
                }
                frame True {
                }
              }
              n594 = case shown="False" w125 {
                tunnel: w124 -> [w365 w369]
                tunnel: [w367 w369] -> w123
                tunnel: [w364 w369] -> w122
                frame False {
                  n595 = Multiply(x=w365, y=0.5) -> (x*y=w367:dbl)
                  n596 = Multiply(x=w365, y=0.2) -> (x*y=w364:dbl)
                }
                frame True {
                }
              }
              n597 = case shown="False" w121 {
                tunnel: w120 -> [w359 w363]
                tunnel: [w361 w363] -> w119
                tunnel: [w358 w363] -> w118
                frame False {
                  n598 = Multiply(x=w359, y=0.5) -> (x*y=w361:dbl)
                  n599 = Multiply(x=w359, y=0.2) -> (x*y=w358:dbl)
                }
                frame True {
                }
              }
              n600 = case shown="False" w117 {
                tunnel: w116 -> [w353 w357]
                tunnel: [w355 w357] -> w115
                tunnel: [w352 w357] -> w114
                frame False {
                  n601 = Multiply(x=w353, y=0.5) -> (x*y=w355:dbl)
                  n602 = Multiply(x=w353, y=0.2) -> (x*y=w352:dbl)
                }
                frame True {
                }
              }
              n603 = case shown="False" w113 {
                tunnel: w112 -> [w347 w351]
                tunnel: [w349 w351] -> w111
                tunnel: [w346 w351] -> w110
                frame False {
                  n604 = Multiply(x=w347, y=0.5) -> (x*y=w349:dbl)
                  n605 = Multiply(x=w347, y=0.2) -> (x*y=w346:dbl)
                }
                frame True {
                }
              }
              n606 = case shown="False" w109 {
                tunnel: w108 -> [w341 w345]
                tunnel: [w343 w345] -> w106
                tunnel: [w340 w345] -> w107
                frame False {
                  n607 = Multiply(x=w341, y=0.5) -> (x*y=w343:dbl)
                  n608 = Multiply(x=w341, y=0.2) -> (x*y=w340:dbl)
                }
                frame True {
                }
              }
              n609 = case shown="False" w105 {
                tunnel: w104 -> [w335 w339]
                tunnel: [w337 w339] -> w103
                tunnel: [w334 w339] -> w102
                frame False {
                  n610 = Multiply(x=w335, y=0.5) -> (x*y=w337:dbl)
                  n611 = Multiply(x=w335, y=0.2) -> (x*y=w334:dbl)
                }
                frame True {
                }
              }
              n612 = case shown="False" w100 {
                tunnel: w101 -> [w329 w333]
                tunnel: [w331 w333] -> w99
                tunnel: [w328 w333] -> w98
                frame False {
                  n613 = Multiply(x=w329, y=0.5) -> (x*y=w331:dbl)
                  n614 = Multiply(x=w329, y=0.2) -> (x*y=w328:dbl)
                }
                frame True {
                }
              }
              n615 = case shown="False" w96 {
                tunnel: w97 -> [w323 w327]
                tunnel: [w325 w327] -> w95
                tunnel: [w322 w327] -> w94
                frame False {
                  n616 = Multiply(x=w323, y=0.5) -> (x*y=w325:dbl)
                  n617 = Multiply(x=w323, y=0.2) -> (x*y=w322:dbl)
                }
                frame True {
                }
              }
              n618 = case shown="False" w92 {
                tunnel: w93 -> [w317 w321]
                tunnel: [w319 w321] -> w91
                tunnel: [w316 w321] -> w90
                frame False {
                  n619 = Multiply(x=w317, y=0.5) -> (x*y=w319:dbl)
                  n620 = Multiply(x=w317, y=0.2) -> (x*y=w316:dbl)
                }
                frame True {
                }
              }
              n621 = case shown="False" w88 {
                tunnel: w89 -> [w311 w315]
                tunnel: [w313 w315] -> w86
                tunnel: [w310 w315] -> w87
                frame False {
                  n622 = Multiply(x=w311, y=0.5) -> (x*y=w313:dbl)
                  n623 = Multiply(x=w311, y=0.2) -> (x*y=w310:dbl)
                }
                frame True {
                }
              }
              n624 = case shown="False" w84 {
                tunnel: w85 -> [w305 w309]
                tunnel: [w307 w309] -> w83
                tunnel: [w304 w309] -> w82
                frame False {
                  n625 = Multiply(x=w305, y=0.5) -> (x*y=w307:dbl)
                  n626 = Multiply(x=w305, y=0.2) -> (x*y=w304:dbl)
                }
                frame True {
                }
              }
              n627 = case shown="False" w80 {
                tunnel: w81 -> [w299 w303]
                tunnel: [w301 w303] -> w79
                tunnel: [w298 w303] -> w78
                frame False {
                  n628 = Multiply(x=w299, y=0.5) -> (x*y=w301:dbl)
                  n629 = Multiply(x=w299, y=0.2) -> (x*y=w298:dbl)
                }
                frame True {
                }
              }
              n630 = case shown="False" w75 {
                tunnel: w74 -> [w293 w297]
                tunnel: [w295 w297] -> w77
                tunnel: [w292 w297] -> w76
                frame False {
                  n631 = Multiply(x=w293, y=0.5) -> (x*y=w295:dbl)
                  n632 = Multiply(x=w293, y=0.2) -> (x*y=w292:dbl)
                }
                frame True {
                }
              }
              n633 = case shown="False" w72 {
                tunnel: w73 -> [w287 w291]
                tunnel: [w289 w291] -> w71
                tunnel: [w286 w291] -> w70
                frame False {
                  n634 = Multiply(x=w287, y=0.5) -> (x*y=w289:dbl)
                  n635 = Multiply(x=w287, y=0.2) -> (x*y=w286:dbl)
                }
                frame True {
                }
              }
              n636 = call "Spänning-till-intensitet v0.4.vi"("Spänning"=w138) -> ("Intensitet"=w136:dbl[])
              n637 = call "Intensitet-till-procent v0.4.vi"("intensitet"=w136) -> ("procent"=w137:dbl[])
              n638 = case shown="0, 2..5, Default" "Alternativ" {
                tunnel: w137 -> [_ w395]
                frame 1 {
                  w378 = T2."Enabled" ("Disabled")
                  # "Vid fallet då reglagen anger intensiteten aktiveras de."
                  n639 = property on="Reglage 660 nm" class="Slide (strict)"("DisabledEnum"=w378) -> ()  [unwired: 2 in, 2 out]
                  n640 = property on="Reglage 520 nm" class="Slide (strict)"("DisabledEnum"=w378) -> ()  [unwired: 2 in, 2 out]
                  n641 = property on="Reglage 750 nm" class="Slide (strict)"("DisabledEnum"=w378) -> ()  [unwired: 2 in, 2 out]
                  n642 = property on="Reglage 490 nm" class="Slide (strict)"("DisabledEnum"=w378) -> ()  [unwired: 2 in, 2 out]
                  n643 = property on="Reglage 515 nm" class="Slide (strict)"("DisabledEnum"=w378) -> ()  [unwired: 2 in, 2 out]
                  n644 = property on="Reglage 590 nm" class="Slide (strict)"("DisabledEnum"=w378) -> ()  [unwired: 2 in, 2 out]
                  n645 = property on="Reglage 420 nm" class="Slide (strict)"("DisabledEnum"=w378) -> ()  [unwired: 2 in, 2 out]
                  n646 = property on="Reglage 945 nm" class="Slide (strict)"("DisabledEnum"=w378) -> ()  [unwired: 2 in, 2 out]
                  n647 = property on="Reglage 830 nm" class="Slide (strict)"("DisabledEnum"=w378) -> ()  [unwired: 2 in, 2 out]
                  n648 = property on="Reglage 880 nm" class="Slide (strict)"("DisabledEnum"=w378) -> ()  [unwired: 2 in, 2 out]
                  n649 = property on="Reglage 450 nm" class="Slide (strict)"("DisabledEnum"=w378) -> ()  [unwired: 2 in, 2 out]
                  n650 = property on="Reglage 980 nm" class="Slide (strict)"("DisabledEnum"=w378) -> ()  [unwired: 2 in, 2 out]
                  n651 = property on="Reglage 780 nm" class="Slide (strict)"("DisabledEnum"=w378) -> ()  [unwired: 2 in, 2 out]
                  n652 = property on="Reglage 720 nm" class="Slide (strict)"("DisabledEnum"=w378) -> ()  [unwired: 2 in, 2 out]
                  n653 = property on="Reglage 630 nm" class="Slide (strict)"("DisabledEnum"=w378) -> ()  [unwired: 2 in, 2 out]
                  n654 = property on="Reglage 680 nm" class="Slide (strict)"("DisabledEnum"=w378) -> ()  [unwired: 2 in, 2 out]
                }
                frame 0, 2..5, Default {
                  w396 = T2."Disabled and Grayed Out" ("Disabled")
                  # "I alla de fall då inte intensiteterna väljs med reglagen\ninaktiveras de medan intensiteterna skrivs ut på dem."
                  n655 = Index Array(array=w395) -> (element #1=w394:dbl, element #2=w393:dbl, element #3=w392:dbl, element #4=w391:dbl, element #5=w390:dbl, element #6=w389:dbl, element #7=w388:dbl, element #8=w387:dbl, element #9=w386:dbl, element #10=w385:dbl, element #11=w384:dbl, element #12=w383:dbl, element #13=w382:dbl, element #14=w381:dbl, element #15=w380:dbl, element #16=w379:dbl)  [unwired: 16 in]
                  n656 = local write "Reglage 520 nm"(w394) -> ()
                  n657 = local write "Reglage 680 nm"(w393) -> ()
                  n658 = local write "Reglage 945 nm"(w392) -> ()
                  n659 = local write "Reglage 880 nm"(w391) -> ()
                  n660 = local write "Reglage 420 nm"(w390) -> ()
                  n661 = local write "Reglage 450 nm"(w389) -> ()
                  n662 = local write "Reglage 780 nm"(w388) -> ()
                  n663 = local write "Reglage 630 nm"(w387) -> ()
                  n664 = local write "Reglage 660 nm"(w386) -> ()
                  n665 = local write "Reglage 750 nm"(w385) -> ()
                  n666 = local write "Reglage 490 nm"(w384) -> ()
                  n667 = local write "Reglage 515 nm"(w383) -> ()
                  n668 = local write "Reglage 590 nm"(w382) -> ()
                  n669 = local write "Reglage 830 nm"(w381) -> ()
                  n670 = local write "Reglage 980 nm"(w380) -> ()
                  n671 = local write "Reglage 720 nm"(w379) -> ()
                  n672 = property on="Reglage 660 nm" class="Slide (strict)"("DisabledEnum"=w396) -> ()  [unwired: 2 in, 2 out]
                  n673 = property on="Reglage 680 nm" class="Slide (strict)"("DisabledEnum"=w396) -> ()  [unwired: 2 in, 2 out]
                  n674 = property on="Reglage 750 nm" class="Slide (strict)"("DisabledEnum"=w396) -> ()  [unwired: 2 in, 2 out]
                  n675 = property on="Reglage 490 nm" class="Slide (strict)"("DisabledEnum"=w396) -> ()  [unwired: 2 in, 2 out]
                  n676 = property on="Reglage 515 nm" class="Slide (strict)"("DisabledEnum"=w396) -> ()  [unwired: 2 in, 2 out]
                  n677 = property on="Reglage 590 nm" class="Slide (strict)"("DisabledEnum"=w396) -> ()  [unwired: 2 in, 2 out]
                  n678 = property on="Reglage 420 nm" class="Slide (strict)"("DisabledEnum"=w396) -> ()  [unwired: 2 in, 2 out]
                  n679 = property on="Reglage 830 nm" class="Slide (strict)"("DisabledEnum"=w396) -> ()  [unwired: 2 in, 2 out]
                  n680 = property on="Reglage 450 nm" class="Slide (strict)"("DisabledEnum"=w396) -> ()  [unwired: 2 in, 2 out]
                  n681 = property on="Reglage 780 nm" class="Slide (strict)"("DisabledEnum"=w396) -> ()  [unwired: 2 in, 2 out]
                  n682 = property on="Reglage 945 nm" class="Slide (strict)"("DisabledEnum"=w396) -> ()  [unwired: 2 in, 2 out]
                  n683 = property on="Reglage 720 nm" class="Slide (strict)"("DisabledEnum"=w396) -> ()  [unwired: 2 in, 2 out]
                  n684 = property on="Reglage 880 nm" class="Slide (strict)"("DisabledEnum"=w396) -> ()  [unwired: 2 in, 2 out]
                  n685 = property on="Reglage 630 nm" class="Slide (strict)"("DisabledEnum"=w396) -> ()  [unwired: 2 in, 2 out]
                  n686 = property on="Reglage 980 nm" class="Slide (strict)"("DisabledEnum"=w396) -> ()  [unwired: 2 in, 2 out]
                  n687 = property on="Reglage 520 nm" class="Slide (strict)"("DisabledEnum"=w396) -> ()  [unwired: 2 in, 2 out]
                }
              }
              n688 = local read "Tänd/släck solen"() -> (w176:bool)
              n689 = call "Simulate Signal"("Offset"=w177, "Frequency"="Frekvens (520 nm)", "Amplitude"=w130) -> ("Sine"=w193:dynamicdata)  [unwired: 11 in, 1 out]
              n690 = call "Simulate Signal2"("Offset"=w127, "Frequency"="Frekvens (680 nm)", "Amplitude"=w126) -> ("Sine"=w192:dynamicdata)  [unwired: 11 in, 1 out]
              n691 = call "Simulate Signal3"("Offset"=w123, "Frequency"="Frekvens (945 nm)", "Amplitude"=w122) -> ("Sine"=w184:dynamicdata)  [unwired: 11 in, 1 out]
              n692 = call "Simulate Signal4"("Offset"=w119, "Frequency"="Frekvens (880 nm)", "Amplitude"=w118) -> ("Sine"=w180:dynamicdata)  [unwired: 11 in, 1 out]
              n693 = call "Simulate Signal5"("Offset"=w115, "Frequency"="Frekvens (420 nm)", "Amplitude"=w114) -> ("Sine"=w189:dynamicdata)  [unwired: 11 in, 1 out]
              n694 = call "Simulate Signal6"("Offset"=w111, "Frequency"="Frekvens (450 nm)", "Amplitude"=w110) -> ("Sine"=w183:dynamicdata)  [unwired: 11 in, 1 out]
              n695 = call "Simulate Signal7"("Offset"=w106, "Frequency"="Frekvens (780 nm)", "Amplitude"=w107) -> ("Sine"=w190:dynamicdata)  [unwired: 11 in, 1 out]
              n696 = call "Simulate Signal8"("Offset"=w103, "Frequency"="Frekvens (630 nm)", "Amplitude"=w102) -> ("Sine"=w182:dynamicdata)  [unwired: 11 in, 1 out]
              n697 = call "Simulate Signal9"("Offset"=w99, "Frequency"="Frekvens (660 nm)", "Amplitude"=w98) -> ("Sine"=w186:dynamicdata)  [unwired: 11 in, 1 out]
              n698 = call "Simulate Signal10"("Offset"=w95, "Frequency"="Frekvens (750 nm)", "Amplitude"=w94) -> ("Sine"=w185:dynamicdata)  [unwired: 11 in, 1 out]
              n699 = call "Simulate Signal11"("Offset"=w91, "Frequency"="Frekvens (490 nm)", "Amplitude"=w90) -> ("Sine"=w179:dynamicdata)  [unwired: 11 in, 1 out]
              n700 = call "Simulate Signal12"("Offset"=w86, "Frequency"="Frekvens (515 nm)", "Amplitude"=w87) -> ("Sine"=w178:dynamicdata)  [unwired: 11 in, 1 out]
              n701 = call "Simulate Signal13"("Offset"=w83, "Frequency"="Frekvens (590 nm)", "Amplitude"=w82) -> ("Sine"=w191:dynamicdata)  [unwired: 11 in, 1 out]
              n702 = call "Simulate Signal14"("Offset"=w79, "Frequency"="Frekvens (830 nm)", "Amplitude"=w78) -> ("Sine"=w187:dynamicdata)  [unwired: 11 in, 1 out]
              n703 = call "Simulate Signal15"("Offset"=w77, "Frequency"="Frekvens (980 nm)", "Amplitude"=w76) -> ("Sine"=w181:dynamicdata)  [unwired: 11 in, 1 out]
              n704 = call "Simulate Signal16"("Offset"=w71, "Frequency"="Frekvens (720 nm)", "Amplitude"=w70) -> ("Sine"=w188:dynamicdata)  [unwired: 11 in, 1 out]
              n705 = Not(x=w176) -> (.not. x?=w149:bool)
              n706 = Merge Signals(w193, w192, w184, w180, w189, w183, w190, w182, w186, w185, w179, w178, w191, w187, w181, w188) -> (w145:dynamicdata)
              n707 = call "DAQ Assistant"("data"=w145, "stop (F)"=w149) -> ("stopped"=w150:bool, "error out"=w144:errorcluster)  [unwired: 15 in, 1 out]
            }
            n708 = call-poly <vilib>:"DAQmx Write.vi"("task/channels in"=refnum<k21> "MyVoltageOutTask_2", "data"=dbl[] [0.0, 0.0, 0.0, 0.0, 0.0, 0.0, 0.0, 0.0, 0.0, 0.0, 0.0, 0.0, 0.0, 0.0, 0.0, 0.0], "error in"=w28) -> ()  [unwired: 10 in, 3 out]
          }
        }
      }
    }
    n709 = local read "Tänd/släck solen"() -> (w15:bool)
    n710 = Not(x=w15) -> (.not. x?=w16:bool)
    n711 = And(x=w16, y="Avsluta programmet") -> (x .and. y?=w14:bool)
    n712 = case shown="True" w14 {
      frame False {
      }
      frame True {
        n713 = Two Button Dialog(message="Är du säker på att du vill avsluta?", 1:"Nej, jag vill fortsätta sola." ("F button name (\"Cancel\")"), 2:"Ja" ("T button name (\"OK\")")) -> (T button?=w19:bool)
        n714 = case shown="True" w19 {
          frame False {
            w21 = FALSE ("EQE-mätning")
            n715 = local write "Avsluta programmet"(w21) -> ()
            n716 = local write "stop"(w21) -> ()
          }
          frame True {
            n717 = local write "Avsluta programmet"(FALSE ("EQE-mätning")) -> ()
            n718 = local write "stop"(TRUE ("Avsluta programmet")) -> ()
          }
        }
      }
    }
  }
  "EQEvarv" <- 0 ("EQEvarv")
  "EQEvarv 2" <- 0 ("EQEvarv 2")
